vi "EOL Vent AP Test.vi"(7 "scaling factor":dbl=11.1, 10 "input cluster":T2 {"LIN INFO"."NAD" format="%.0x"; "LIN INFO"."ADCS LIN"."HW select" items=["NI-XNET", "NI-CAN"]; "LVDT Status"."LVDT's stored config"."Lower Limit" format="%.2f"; "LVDT Status"."LVDT's stored config"."Upper Limit" format="%.2f"; "PLC Comms"."PLC string write Tags"."error message 9"."DataSocket Reference"."OnStatusUpdated" format="%.0x"; "PLC Comms"."PLC string write Tags"."error message 9"."DataSocket Reference"."OnDataUpdated" format="%.0x"; "PLC Comms"."PLC string write Tags"."error message 8"."DataSocket Reference"."OnStatusUpdated" format="%.0x"; "PLC Comms"."PLC string write Tags"."error message 8"."DataSocket Reference"."OnDataUpdated" format="%.0x"; "PLC Comms"."PLC string write Tags"."error message 7"."DataSocket Reference"."OnStatusUpdated" format="%.0x"; "PLC Comms"."PLC string write Tags"."error message 7"."DataSocket Reference"."OnDataUpdated" format="%.0x"; "PLC Comms"."PLC string write Tags"."error message 6"."DataSocket Reference"."OnStatusUpdated" format="%.0x"; "PLC Comms"."PLC string write Tags"."error message 6"."DataSocket Reference"."OnDataUpdated" format="%.0x"; "PLC Comms"."PLC string write Tags"."error message 5"."DataSocket Reference"."OnStatusUpdated" format="%.0x"; "PLC Comms"."PLC string write Tags"."error message 5"."DataSocket Reference"."OnDataUpdated" format="%.0x"; "PLC Comms"."PLC string write Tags"."error message 4"."DataSocket Reference"."OnStatusUpdated" format="%.0x"; "PLC Comms"."PLC string write Tags"."error message 4"."DataSocket Reference"."OnDataUpdated" format="%.0x"; "PLC Comms"."PLC string write Tags"."error message 3"."DataSocket Reference"."OnStatusUpdated" format="%.0x"; "PLC Comms"."PLC string write Tags"."error message 3"."DataSocket Reference"."OnDataUpdated" format="%.0x"; "PLC Comms"."PLC string write Tags"."error message 2"."DataSocket Reference"."OnStatusUpdated" format="%.0x"; "PLC Comms"."PLC string write Tags"."error message 2"."DataSocket Reference"."OnDataUpdated" format="%.0x"; "PLC Comms"."PLC string write Tags"."error message 1"."DataSocket Reference"."OnStatusUpdated" format="%.0x"; "PLC Comms"."PLC string write Tags"."error message 1"."DataSocket Reference"."OnDataUpdated" format="%.0x"; "PLC Comms"."PLC string write Tags"."error message 0"."DataSocket Reference"."OnStatusUpdated" format="%.0x"; "PLC Comms"."PLC string write Tags"."error message 0"."DataSocket Reference"."OnDataUpdated" format="%.0x"; "PLC Comms"."PLC string write Tags"."barcode station error"."DataSocket Reference"."OnStatusUpdated" format="%.0x"; "PLC Comms"."PLC string write Tags"."barcode station error"."DataSocket Reference"."OnDataUpdated" format="%.0x"; "PLC Comms"."PLC string read Tags"."iGPS SN 9"."DataSocket Reference"."OnStatusUpdated" format="%.0x"; "PLC Comms"."PLC string read Tags"."iGPS SN 9"."DataSocket Reference"."OnDataUpdated" format="%.0x"; "PLC Comms"."PLC string read Tags"."iGPS SN 8"."DataSocket Reference"."OnStatusUpdated" format="%.0x"; "PLC Comms"."PLC string read Tags"."iGPS SN 8"."DataSocket Reference"."OnDataUpdated" format="%.0x"; "PLC Comms"."PLC string read Tags"."iGPS SN 7"."DataSocket Reference"."OnStatusUpdated" format="%.0x"; "PLC Comms"."PLC string read Tags"."iGPS SN 7"."DataSocket Reference"."OnDataUpdated" format="%.0x"; "PLC Comms"."PLC string read Tags"."iGPS SN 6"."DataSocket Reference"."OnStatusUpdated" format="%.0x"; "PLC Comms"."PLC string read Tags"."iGPS SN 6"."DataSocket Reference"."OnDataUpdated" format="%.0x"; "PLC Comms"."PLC string read Tags"."iGPS SN 5"."DataSocket Reference"."OnStatusUpdated" format="%.0x"; "PLC Comms"."PLC string read Tags"."iGPS SN 5"."DataSocket Reference"."OnDataUpdated" format="%.0x"; "PLC Comms"."PLC string read Tags"."iGPS SN 4"."DataSocket Reference"."OnStatusUpdated" format="%.0x"; "PLC Comms"."PLC string read Tags"."iGPS SN 4"."DataSocket Reference"."OnDataUpdated" format="%.0x"; "PLC Comms"."PLC string read Tags"."iGPS SN 3"."DataSocket Reference"."OnStatusUpdated" format="%.0x"; "PLC Comms"."PLC string read Tags"."iGPS SN 3"."DataSocket Reference"."OnDataUpdated" format="%.0x"; "PLC Comms"."PLC string read Tags"."iGPS SN 2"."DataSocket Reference"."OnStatusUpdated" format="%.0x"; "PLC Comms"."PLC string read Tags"."iGPS SN 2"."DataSocket Reference"."OnDataUpdated" format="%.0x"; "PLC Comms"."PLC string read Tags"."iGPS SN 1"."DataSocket Reference"."OnStatusUpdated" format="%.0x"; "PLC Comms"."PLC string read Tags"."iGPS SN 1"."DataSocket Reference"."OnDataUpdated" format="%.0x"; "PLC Comms"."PLC string read Tags"."iGPS SN 0"."DataSocket Reference"."OnStatusUpdated" format="%.0x"; "PLC Comms"."PLC string read Tags"."iGPS SN 0"."DataSocket Reference"."OnDataUpdated" format="%.0x"; "PLC Comms"."PLC string read Tags"."Manual Part History Number"."DataSocket Reference"."OnStatusUpdated" format="%.0x"; "PLC Comms"."PLC string read Tags"."Manual Part History Number"."DataSocket Reference"."OnDataUpdated" format="%.0x"; "PLC Comms"."PLC string read Tags"."Manual Customer Number"."DataSocket Reference"."OnStatusUpdated" format="%.0x"; "PLC Comms"."PLC string read Tags"."Manual Customer Number"."DataSocket Reference"."OnDataUpdated" format="%.0x"; "PLC Comms"."PLC string read Tags"."Manual Model Type"."DataSocket Reference"."OnStatusUpdated" format="%.0x"; "PLC Comms"."PLC string read Tags"."Manual Model Type"."DataSocket Reference"."OnDataUpdated" format="%.0x"; "PLC Comms"."PLC string read Tags"."Manual Shade Color"."DataSocket Reference"."OnStatusUpdated" format="%.0x"; "PLC Comms"."PLC string read Tags"."Manual Shade Color"."DataSocket Reference"."OnDataUpdated" format="%.0x"; "PLC Comms"."PLC string read Tags"."Manual Inalfa Part Number"."DataSocket Reference"."OnStatusUpdated" format="%.0x"; "PLC Comms"."PLC string read Tags"."Manual Inalfa Part Number"."DataSocket Reference"."OnDataUpdated" format="%.0x"; "PLC Comms"."PLC string read Tags"."Manual Serial Number"."DataSocket Reference"."OnStatusUpdated" format="%.0x"; "PLC Comms"."PLC string read Tags"."Manual Serial Number"."DataSocket Reference"."OnDataUpdated" format="%.0x"; "PLC Comms"."PLC string read Tags"."Shade 2 Barcode"."DataSocket Reference"."OnStatusUpdated" format="%.0x"; "PLC Comms"."PLC string read Tags"."Shade 2 Barcode"."DataSocket Reference"."OnDataUpdated" format="%.0x"; "PLC Comms"."PLC string read Tags"."Shade 1 Barcode"."DataSocket Reference"."OnStatusUpdated" format="%.0x"; "PLC Comms"."PLC string read Tags"."Shade 1 Barcode"."DataSocket Reference"."OnDataUpdated" format="%.0x"; "PLC Comms"."PLC string read Tags"."Part History Number"."DataSocket Reference"."OnStatusUpdated" format="%.0x"; "PLC Comms"."PLC string read Tags"."Part History Number"."DataSocket Reference"."OnDataUpdated" format="%.0x"; "PLC Comms"."PLC string read Tags"."Customer Number"."DataSocket Reference"."OnStatusUpdated" format="%.0x"; "PLC Comms"."PLC string read Tags"."Customer Number"."DataSocket Reference"."OnDataUpdated" format="%.0x"; "PLC Comms"."PLC string read Tags"."Model Type"."DataSocket Reference"."OnStatusUpdated" format="%.0x"; "PLC Comms"."PLC string read Tags"."Model Type"."DataSocket Reference"."OnDataUpdated" format="%.0x"; "PLC Comms"."PLC string read Tags"."Shade Color"."DataSocket Reference"."OnStatusUpdated" format="%.0x"; "PLC Comms"."PLC string read Tags"."Shade Color"."DataSocket Reference"."OnDataUpdated" format="%.0x"; "PLC Comms"."PLC string read Tags"."Inalfa Part Number"."DataSocket Reference"."OnStatusUpdated" format="%.0x"; "PLC Comms"."PLC string read Tags"."Inalfa Part Number"."DataSocket Reference"."OnDataUpdated" format="%.0x"; "PLC Comms"."PLC string read Tags"."Pallet Number"."DataSocket Reference"."OnStatusUpdated" format="%.0x"; "PLC Comms"."PLC string read Tags"."Pallet Number"."DataSocket Reference"."OnDataUpdated" format="%.0x"; "PLC Comms"."PLC string read Tags"."Serial Number"."DataSocket Reference"."OnStatusUpdated" format="%.0x"; "PLC Comms"."PLC string read Tags"."Serial Number"."DataSocket Reference"."OnDataUpdated" format="%.0x"; "PLC Comms"."PLC bool write Tags"."Move LVDT Adjust Station"."DataSocket Reference"."OnStatusUpdated" format="%.0x"; "PLC Comms"."PLC bool write Tags"."Move LVDT Adjust Station"."DataSocket Reference"."OnDataUpdated" format="%.0x"; "PLC Comms"."PLC bool write Tags"."AT set to Vent ATS Home Pos"."DataSocket Reference"."OnStatusUpdated" format="%.0x"; "PLC Comms"."PLC bool write Tags"."AT set to Vent ATS Home Pos"."DataSocket Reference"."OnDataUpdated" format="%.0x"; "PLC Comms"."PLC bool write Tags"."AT set to Vent ATS Test Pos"."DataSocket Reference"."OnStatusUpdated" format="%.0x"; "PLC Comms"."PLC bool write Tags"."AT set to Vent ATS Test Pos"."DataSocket Reference"."OnDataUpdated" format="%.0x"; "PLC Comms"."PLC bool write Tags"."Barcode02 OK"."DataSocket Reference"."OnStatusUpdated" format="%.0x"; "PLC Comms"."PLC bool write Tags"."Barcode02 OK"."DataSocket Reference"."OnDataUpdated" format="%.0x"; "PLC Comms"."PLC bool write Tags"."Barcode01 OK"."DataSocket Reference"."OnStatusUpdated" format="%.0x"; "PLC Comms"."PLC bool write Tags"."Barcode01 OK"."DataSocket Reference"."OnDataUpdated" format="%.0x"; "PLC Comms"."PLC bool write Tags"."AT set wand 02 home pos"."DataSocket Reference"."OnStatusUpdated" format="%.0x"; "PLC Comms"."PLC bool write Tags"."AT set wand 02 home pos"."DataSocket Reference"."OnDataUpdated" format="%.0x"; "PLC Comms"."PLC bool write Tags"."AT set sunshade 02 wand up"."DataSocket Reference"."OnStatusUpdated" format="%.0x"; "PLC Comms"."PLC bool write Tags"."AT set sunshade 02 wand up"."DataSocket Reference"."OnDataUpdated" format="%.0x"; "PLC Comms"."PLC bool write Tags"."NVH Operator Finish"."DataSocket Reference"."OnStatusUpdated" format="%.0x"; "PLC Comms"."PLC bool write Tags"."NVH Operator Finish"."DataSocket Reference"."OnDataUpdated" format="%.0x"; "PLC Comms"."PLC bool write Tags"."NVH Operator Glass Close Noise"."DataSocket Reference"."OnStatusUpdated" format="%.0x"; "PLC Comms"."PLC bool write Tags"."NVH Operator Glass Close Noise"."DataSocket Reference"."OnDataUpdated" format="%.0x"; "PLC Comms"."PLC bool write Tags"."NVH Operator Glass Open Noise"."DataSocket Reference"."OnStatusUpdated" format="%.0x"; "PLC Comms"."PLC bool write Tags"."NVH Operator Glass Open Noise"."DataSocket Reference"."OnDataUpdated" format="%.0x"; "PLC Comms"."PLC bool write Tags"."NVH Operator Sunshade Close Noise"."DataSocket Reference"."OnStatusUpdated" format="%.0x"; "PLC Comms"."PLC bool write Tags"."NVH Operator Sunshade Close Noise"."DataSocket Reference"."OnDataUpdated" format="%.0x"; "PLC Comms"."PLC bool write Tags"."NVH Operator Sunshade Open Noise"."DataSocket Reference"."OnStatusUpdated" format="%.0x"; "PLC Comms"."PLC bool write Tags"."NVH Operator Sunshade Open Noise"."DataSocket Reference"."OnDataUpdated" format="%.0x"; "PLC Comms"."PLC bool write Tags"."NVH Operator Vent Close Noise"."DataSocket Reference"."OnStatusUpdated" format="%.0x"; "PLC Comms"."PLC bool write Tags"."NVH Operator Vent Close Noise"."DataSocket Reference"."OnDataUpdated" format="%.0x"; "PLC Comms"."PLC bool write Tags"."NVH Operator Vent Open Noise"."DataSocket Reference"."OnStatusUpdated" format="%.0x"; "PLC Comms"."PLC bool write Tags"."NVH Operator Vent Open Noise"."DataSocket Reference"."OnDataUpdated" format="%.0x"; "PLC Comms"."PLC bool write Tags"."NVH Operator Check"."DataSocket Reference"."OnStatusUpdated" format="%.0x"; "PLC Comms"."PLC bool write Tags"."NVH Operator Check"."DataSocket Reference"."OnDataUpdated" format="%.0x"; "PLC Comms"."PLC bool write Tags"."NVH Operator Fail"."DataSocket Reference"."OnStatusUpdated" format="%.0x"; "PLC Comms"."PLC bool write Tags"."NVH Operator Fail"."DataSocket Reference"."OnDataUpdated" format="%.0x"; "PLC Comms"."PLC bool write Tags"."NVH Operator Pass"."DataSocket Reference"."OnStatusUpdated" format="%.0x"; "PLC Comms"."PLC bool write Tags"."NVH Operator Pass"."DataSocket Reference"."OnDataUpdated" format="%.0x"; "PLC Comms"."PLC bool write Tags"."NVH Operator Express Rollo Opened02"."DataSocket Reference"."OnStatusUpdated" format="%.0x"; "PLC Comms"."PLC bool write Tags"."NVH Operator Express Rollo Opened02"."DataSocket Reference"."OnDataUpdated" format="%.0x"; "PLC Comms"."PLC bool write Tags"."NVH Operator Express Rollo Closed01"."DataSocket Reference"."OnStatusUpdated" format="%.0x"; "PLC Comms"."PLC bool write Tags"."NVH Operator Express Rollo Closed01"."DataSocket Reference"."OnDataUpdated" format="%.0x"; "PLC Comms"."PLC bool write Tags"."NVH Operator Express Rollo Opened01"."DataSocket Reference"."OnStatusUpdated" format="%.0x"; "PLC Comms"."PLC bool write Tags"."NVH Operator Express Rollo Opened01"."DataSocket Reference"."OnDataUpdated" format="%.0x"; "PLC Comms"."PLC bool write Tags"."NVH Operator Express Glass Closed"."DataSocket Reference"."OnStatusUpdated" format="%.0x"; "PLC Comms"."PLC bool write Tags"."NVH Operator Express Glass Closed"."DataSocket Reference"."OnDataUpdated" format="%.0x"; "PLC Comms"."PLC bool write Tags"."NVH Operator Express Glass Opened"."DataSocket Reference"."OnStatusUpdated" format="%.0x"; "PLC Comms"."PLC bool write Tags"."NVH Operator Express Glass Opened"."DataSocket Reference"."OnDataUpdated" format="%.0x"; "PLC Comms"."PLC bool write Tags"."NVH Fail"."DataSocket Reference"."OnStatusUpdated" format="%.0x"; "PLC Comms"."PLC bool write Tags"."NVH Fail"."DataSocket Reference"."OnDataUpdated" format="%.0x"; "PLC Comms"."PLC bool write Tags"."NVH Pass"."DataSocket Reference"."OnStatusUpdated" format="%.0x"; "PLC Comms"."PLC bool write Tags"."NVH Pass"."DataSocket Reference"."OnDataUpdated" format="%.0x"; "PLC Comms"."PLC bool write Tags"."NVH SunRoof Stop"."DataSocket Reference"."OnStatusUpdated" format="%.0x"; "PLC Comms"."PLC bool write Tags"."NVH SunRoof Stop"."DataSocket Reference"."OnDataUpdated" format="%.0x"; "PLC Comms"."PLC bool write Tags"."NVH SunRoof Moving"."DataSocket Reference"."OnStatusUpdated" format="%.0x"; "PLC Comms"."PLC bool write Tags"."NVH SunRoof Moving"."DataSocket Reference"."OnDataUpdated" format="%.0x"; "PLC Comms"."PLC bool write Tags"."Extend Z LVDTS"."DataSocket Reference"."OnStatusUpdated" format="%.0x"; "PLC Comms"."PLC bool write Tags"."Extend Z LVDTS"."DataSocket Reference"."OnDataUpdated" format="%.0x"; "PLC Comms"."PLC bool write Tags"."Bad Frame Barcode"."DataSocket Reference"."OnStatusUpdated" format="%.0x"; "PLC Comms"."PLC bool write Tags"."Bad Frame Barcode"."DataSocket Reference"."OnDataUpdated" format="%.0x"; "PLC Comms"."PLC bool write Tags"."Good Frame Barcode"."DataSocket Reference"."OnStatusUpdated" format="%.0x"; "PLC Comms"."PLC bool write Tags"."Good Frame Barcode"."DataSocket Reference"."OnDataUpdated" format="%.0x"; "PLC Comms"."PLC bool write Tags"."AT VentPMACExtended"."DataSocket Reference"."OnStatusUpdated" format="%.0x"; "PLC Comms"."PLC bool write Tags"."AT VentPMACExtended"."DataSocket Reference"."OnDataUpdated" format="%.0x"; "PLC Comms"."PLC bool write Tags"."AT VentPMACHome"."DataSocket Reference"."OnStatusUpdated" format="%.0x"; "PLC Comms"."PLC bool write Tags"."AT VentPMACHome"."DataSocket Reference"."OnDataUpdated" format="%.0x"; "PLC Comms"."PLC bool write Tags"."control slide stop"."DataSocket Reference"."OnStatusUpdated" format="%.0x"; "PLC Comms"."PLC bool write Tags"."control slide stop"."DataSocket Reference"."OnDataUpdated" format="%.0x"; "PLC Comms"."PLC bool write Tags"."control slide start"."DataSocket Reference"."OnStatusUpdated" format="%.0x"; "PLC Comms"."PLC bool write Tags"."control slide start"."DataSocket Reference"."OnDataUpdated" format="%.0x"; "PLC Comms"."PLC bool write Tags"."ss servo close"."DataSocket Reference"."OnStatusUpdated" format="%.0x"; "PLC Comms"."PLC bool write Tags"."ss servo close"."DataSocket Reference"."OnDataUpdated" format="%.0x"; "PLC Comms"."PLC bool write Tags"."ss servo open"."DataSocket Reference"."OnStatusUpdated" format="%.0x"; "PLC Comms"."PLC bool write Tags"."ss servo open"."DataSocket Reference"."OnDataUpdated" format="%.0x"; "PLC Comms"."PLC bool write Tags"."Extend LVDT's"."DataSocket Reference"."OnStatusUpdated" format="%.0x"; "PLC Comms"."PLC bool write Tags"."Extend LVDT's"."DataSocket Reference"."OnDataUpdated" format="%.0x"; "PLC Comms"."PLC bool write Tags"."Retract LVDT's"."DataSocket Reference"."OnStatusUpdated" format="%.0x"; "PLC Comms"."PLC bool write Tags"."Retract LVDT's"."DataSocket Reference"."OnDataUpdated" format="%.0x"; "PLC Comms"."PLC bool write Tags"."Test Started"."DataSocket Reference"."OnStatusUpdated" format="%.0x"; "PLC Comms"."PLC bool write Tags"."Test Started"."DataSocket Reference"."OnDataUpdated" format="%.0x"; "PLC Comms"."PLC bool write Tags"."Test Complete Fail"."DataSocket Reference"."OnStatusUpdated" format="%.0x"; "PLC Comms"."PLC bool write Tags"."Test Complete Fail"."DataSocket Reference"."OnDataUpdated" format="%.0x"; "PLC Comms"."PLC bool write Tags"."Test Complete Pass"."DataSocket Reference"."OnStatusUpdated" format="%.0x"; "PLC Comms"."PLC bool write Tags"."Test Complete Pass"."DataSocket Reference"."OnDataUpdated" format="%.0x"; "PLC Comms"."PLC bool write Tags"."AT set wand home pos"."DataSocket Reference"."OnStatusUpdated" format="%.0x"; "PLC Comms"."PLC bool write Tags"."AT set wand home pos"."DataSocket Reference"."OnDataUpdated" format="%.0x"; "PLC Comms"."PLC bool write Tags"."AT set sunshade wand lower"."DataSocket Reference"."OnStatusUpdated" format="%.0x"; "PLC Comms"."PLC bool write Tags"."AT set sunshade wand lower"."DataSocket Reference"."OnDataUpdated" format="%.0x"; "PLC Comms"."PLC bool write Tags"."AT set glass wand lower"."DataSocket Reference"."OnStatusUpdated" format="%.0x"; "PLC Comms"."PLC bool write Tags"."AT set glass wand lower"."DataSocket Reference"."OnDataUpdated" format="%.0x"; "PLC Comms"."PLC boolean read Tags"."Finish Adjust LVDT"."DataSocket Reference"."OnStatusUpdated" format="%.0x"; "PLC Comms"."PLC boolean read Tags"."Finish Adjust LVDT"."DataSocket Reference"."OnDataUpdated" format="%.0x"; "PLC Comms"."PLC boolean read Tags"."Start Adjust LVDT"."DataSocket Reference"."OnStatusUpdated" format="%.0x"; "PLC Comms"."PLC boolean read Tags"."Start Adjust LVDT"."DataSocket Reference"."OnDataUpdated" format="%.0x"; "PLC Comms"."PLC boolean read Tags"."AT at vent ATS Home pos"."DataSocket Reference"."OnStatusUpdated" format="%.0x"; "PLC Comms"."PLC boolean read Tags"."AT at vent ATS Home pos"."DataSocket Reference"."OnDataUpdated" format="%.0x"; "PLC Comms"."PLC boolean read Tags"."AT at vent ATS test pos"."DataSocket Reference"."OnStatusUpdated" format="%.0x"; "PLC Comms"."PLC boolean read Tags"."AT at vent ATS test pos"."DataSocket Reference"."OnDataUpdated" format="%.0x"; "PLC Comms"."PLC boolean read Tags"."NVH Operator Re-do"."DataSocket Reference"."OnStatusUpdated" format="%.0x"; "PLC Comms"."PLC boolean read Tags"."NVH Operator Re-do"."DataSocket Reference"."OnDataUpdated" format="%.0x"; "PLC Comms"."PLC boolean read Tags"."NVH Operator Express Glass Vent Close"."DataSocket Reference"."OnStatusUpdated" format="%.0x"; "PLC Comms"."PLC boolean read Tags"."NVH Operator Express Glass Vent Close"."DataSocket Reference"."OnDataUpdated" format="%.0x"; "PLC Comms"."PLC boolean read Tags"."NVH Operator Express Glass vent Open"."DataSocket Reference"."OnStatusUpdated" format="%.0x"; "PLC Comms"."PLC boolean read Tags"."NVH Operator Express Glass vent Open"."DataSocket Reference"."OnDataUpdated" format="%.0x"; "PLC Comms"."PLC boolean read Tags"."windproof position"."DataSocket Reference"."OnStatusUpdated" format="%.0x"; "PLC Comms"."PLC boolean read Tags"."windproof position"."DataSocket Reference"."OnDataUpdated" format="%.0x"; "PLC Comms"."PLC boolean read Tags"."AT in wand 02 home pos"."DataSocket Reference"."OnStatusUpdated" format="%.0x"; "PLC Comms"."PLC boolean read Tags"."AT in wand 02 home pos"."DataSocket Reference"."OnDataUpdated" format="%.0x"; "PLC Comms"."PLC boolean read Tags"."AT in sunshad 02 wand up pos"."DataSocket Reference"."OnStatusUpdated" format="%.0x"; "PLC Comms"."PLC boolean read Tags"."AT in sunshad 02 wand up pos"."DataSocket Reference"."OnDataUpdated" format="%.0x"; "PLC Comms"."PLC boolean read Tags"."AT shade 02 position"."DataSocket Reference"."OnStatusUpdated" format="%.0x"; "PLC Comms"."PLC boolean read Tags"."AT shade 02 position"."DataSocket Reference"."OnDataUpdated" format="%.0x"; "PLC Comms"."PLC boolean read Tags"."NVH Operator Check"."DataSocket Reference"."OnStatusUpdated" format="%.0x"; "PLC Comms"."PLC boolean read Tags"."NVH Operator Check"."DataSocket Reference"."OnDataUpdated" format="%.0x"; "PLC Comms"."PLC boolean read Tags"."NVH Operator Finish"."DataSocket Reference"."OnStatusUpdated" format="%.0x"; "PLC Comms"."PLC boolean read Tags"."NVH Operator Finish"."DataSocket Reference"."OnDataUpdated" format="%.0x"; "PLC Comms"."PLC boolean read Tags"."NVH Operator Glass Close Noise"."DataSocket Reference"."OnStatusUpdated" format="%.0x"; "PLC Comms"."PLC boolean read Tags"."NVH Operator Glass Close Noise"."DataSocket Reference"."OnDataUpdated" format="%.0x"; "PLC Comms"."PLC boolean read Tags"."NVH Operator Glass Open Noise"."DataSocket Reference"."OnStatusUpdated" format="%.0x"; "PLC Comms"."PLC boolean read Tags"."NVH Operator Glass Open Noise"."DataSocket Reference"."OnDataUpdated" format="%.0x"; "PLC Comms"."PLC boolean read Tags"."NVH Operator Sunshade Close Noise"."DataSocket Reference"."OnStatusUpdated" format="%.0x"; "PLC Comms"."PLC boolean read Tags"."NVH Operator Sunshade Close Noise"."DataSocket Reference"."OnDataUpdated" format="%.0x"; "PLC Comms"."PLC boolean read Tags"."NVH Operator Sunshade Open Noise"."DataSocket Reference"."OnStatusUpdated" format="%.0x"; "PLC Comms"."PLC boolean read Tags"."NVH Operator Sunshade Open Noise"."DataSocket Reference"."OnDataUpdated" format="%.0x"; "PLC Comms"."PLC boolean read Tags"."NVH Operator Vent Close Noise"."DataSocket Reference"."OnStatusUpdated" format="%.0x"; "PLC Comms"."PLC boolean read Tags"."NVH Operator Vent Close Noise"."DataSocket Reference"."OnDataUpdated" format="%.0x"; "PLC Comms"."PLC boolean read Tags"."NVH Operator Vent Open Noise"."DataSocket Reference"."OnStatusUpdated" format="%.0x"; "PLC Comms"."PLC boolean read Tags"."NVH Operator Vent Open Noise"."DataSocket Reference"."OnDataUpdated" format="%.0x"; "PLC Comms"."PLC boolean read Tags"."NVH Operator Express Rollo Close02"."DataSocket Reference"."OnStatusUpdated" format="%.0x"; "PLC Comms"."PLC boolean read Tags"."NVH Operator Express Rollo Close02"."DataSocket Reference"."OnDataUpdated" format="%.0x"; "PLC Comms"."PLC boolean read Tags"."NVH Operator Express Rollo Open02"."DataSocket Reference"."OnStatusUpdated" format="%.0x"; "PLC Comms"."PLC boolean read Tags"."NVH Operator Express Rollo Open02"."DataSocket Reference"."OnDataUpdated" format="%.0x"; "PLC Comms"."PLC boolean read Tags"."NVH Operator Express Rollo Close01"."DataSocket Reference"."OnStatusUpdated" format="%.0x"; "PLC Comms"."PLC boolean read Tags"."NVH Operator Express Rollo Close01"."DataSocket Reference"."OnDataUpdated" format="%.0x"; "PLC Comms"."PLC boolean read Tags"."NVH Operator Express Rollo Open01"."DataSocket Reference"."OnStatusUpdated" format="%.0x"; "PLC Comms"."PLC boolean read Tags"."NVH Operator Express Rollo Open01"."DataSocket Reference"."OnDataUpdated" format="%.0x"; "PLC Comms"."PLC boolean read Tags"."NVH Operator Express Glass Close"."DataSocket Reference"."OnStatusUpdated" format="%.0x"; "PLC Comms"."PLC boolean read Tags"."NVH Operator Express Glass Close"."DataSocket Reference"."OnDataUpdated" format="%.0x"; "PLC Comms"."PLC boolean read Tags"."NVH Operator Express Glass Open"."DataSocket Reference"."OnStatusUpdated" format="%.0x"; "PLC Comms"."PLC boolean read Tags"."NVH Operator Express Glass Open"."DataSocket Reference"."OnDataUpdated" format="%.0x"; "PLC Comms"."PLC boolean read Tags"."NVH Operator Fail"."DataSocket Reference"."OnStatusUpdated" format="%.0x"; "PLC Comms"."PLC boolean read Tags"."NVH Operator Fail"."DataSocket Reference"."OnDataUpdated" format="%.0x"; "PLC Comms"."PLC boolean read Tags"."NVH Operator Pass"."DataSocket Reference"."OnStatusUpdated" format="%.0x"; "PLC Comms"."PLC boolean read Tags"."NVH Operator Pass"."DataSocket Reference"."OnDataUpdated" format="%.0x"; "PLC Comms"."PLC boolean read Tags"."Z LVDTs Extended"."DataSocket Reference"."OnStatusUpdated" format="%.0x"; "PLC Comms"."PLC boolean read Tags"."Z LVDTs Extended"."DataSocket Reference"."OnDataUpdated" format="%.0x"; "PLC Comms"."PLC boolean read Tags"."iGPS Pass 9"."DataSocket Reference"."OnStatusUpdated" format="%.0x"; "PLC Comms"."PLC boolean read Tags"."iGPS Pass 9"."DataSocket Reference"."OnDataUpdated" format="%.0x"; "PLC Comms"."PLC boolean read Tags"."iGPS Pass 8"."DataSocket Reference"."OnStatusUpdated" format="%.0x"; "PLC Comms"."PLC boolean read Tags"."iGPS Pass 8"."DataSocket Reference"."OnDataUpdated" format="%.0x"; "PLC Comms"."PLC boolean read Tags"."iGPS Pass 7"."DataSocket Reference"."OnStatusUpdated" format="%.0x"; "PLC Comms"."PLC boolean read Tags"."iGPS Pass 7"."DataSocket Reference"."OnDataUpdated" format="%.0x"; "PLC Comms"."PLC boolean read Tags"."iGPS Pass 6"."DataSocket Reference"."OnStatusUpdated" format="%.0x"; "PLC Comms"."PLC boolean read Tags"."iGPS Pass 6"."DataSocket Reference"."OnDataUpdated" format="%.0x"; "PLC Comms"."PLC boolean read Tags"."iGPS Pass 5"."DataSocket Reference"."OnStatusUpdated" format="%.0x"; "PLC Comms"."PLC boolean read Tags"."iGPS Pass 5"."DataSocket Reference"."OnDataUpdated" format="%.0x"; "PLC Comms"."PLC boolean read Tags"."iGPS Pass 4"."DataSocket Reference"."OnStatusUpdated" format="%.0x"; "PLC Comms"."PLC boolean read Tags"."iGPS Pass 4"."DataSocket Reference"."OnDataUpdated" format="%.0x"; "PLC Comms"."PLC boolean read Tags"."iGPS Pass 3"."DataSocket Reference"."OnStatusUpdated" format="%.0x"; "PLC Comms"."PLC boolean read Tags"."iGPS Pass 3"."DataSocket Reference"."OnDataUpdated" format="%.0x"; "PLC Comms"."PLC boolean read Tags"."iGPS Pass 2"."DataSocket Reference"."OnStatusUpdated" format="%.0x"; "PLC Comms"."PLC boolean read Tags"."iGPS Pass 2"."DataSocket Reference"."OnDataUpdated" format="%.0x"; "PLC Comms"."PLC boolean read Tags"."iGPS Pass 1"."DataSocket Reference"."OnStatusUpdated" format="%.0x"; "PLC Comms"."PLC boolean read Tags"."iGPS Pass 1"."DataSocket Reference"."OnDataUpdated" format="%.0x"; "PLC Comms"."PLC boolean read Tags"."iGPS Pass 0"."DataSocket Reference"."OnStatusUpdated" format="%.0x"; "PLC Comms"."PLC boolean read Tags"."iGPS Pass 0"."DataSocket Reference"."OnDataUpdated" format="%.0x"; "PLC Comms"."PLC boolean read Tags"."Check Frame Barcode"."DataSocket Reference"."OnStatusUpdated" format="%.0x"; "PLC Comms"."PLC boolean read Tags"."Check Frame Barcode"."DataSocket Reference"."OnDataUpdated" format="%.0x"; "PLC Comms"."PLC boolean read Tags"."SS Barcode Scanner Bypassed"."DataSocket Reference"."OnStatusUpdated" format="%.0x"; "PLC Comms"."PLC boolean read Tags"."SS Barcode Scanner Bypassed"."DataSocket Reference"."OnDataUpdated" format="%.0x"; "PLC Comms"."PLC boolean read Tags"."AT VentPMACisExtend"."DataSocket Reference"."OnStatusUpdated" format="%.0x"; "PLC Comms"."PLC boolean read Tags"."AT VentPMACisExtend"."DataSocket Reference"."OnDataUpdated" format="%.0x"; "PLC Comms"."PLC boolean read Tags"."AT VentPMACatHome"."DataSocket Reference"."OnStatusUpdated" format="%.0x"; "PLC Comms"."PLC boolean read Tags"."AT VentPMACatHome"."DataSocket Reference"."OnDataUpdated" format="%.0x"; "PLC Comms"."PLC boolean read Tags"."wind deflector low speed pos"."DataSocket Reference"."OnStatusUpdated" format="%.0x"; "PLC Comms"."PLC boolean read Tags"."wind deflector low speed pos"."DataSocket Reference"."OnDataUpdated" format="%.0x"; "PLC Comms"."PLC boolean read Tags"."wind deflector high speed pos"."DataSocket Reference"."OnStatusUpdated" format="%.0x"; "PLC Comms"."PLC boolean read Tags"."wind deflector high speed pos"."DataSocket Reference"."OnDataUpdated" format="%.0x"; "PLC Comms"."PLC boolean read Tags"."control slide right over stroke"."DataSocket Reference"."OnStatusUpdated" format="%.0x"; "PLC Comms"."PLC boolean read Tags"."control slide right over stroke"."DataSocket Reference"."OnDataUpdated" format="%.0x"; "PLC Comms"."PLC boolean read Tags"."control slide right good"."DataSocket Reference"."OnStatusUpdated" format="%.0x"; "PLC Comms"."PLC boolean read Tags"."control slide right good"."DataSocket Reference"."OnDataUpdated" format="%.0x"; "PLC Comms"."PLC boolean read Tags"."control slide left over stroke"."DataSocket Reference"."OnStatusUpdated" format="%.0x"; "PLC Comms"."PLC boolean read Tags"."control slide left over stroke"."DataSocket Reference"."OnDataUpdated" format="%.0x"; "PLC Comms"."PLC boolean read Tags"."control slide left good"."DataSocket Reference"."OnStatusUpdated" format="%.0x"; "PLC Comms"."PLC boolean read Tags"."control slide left good"."DataSocket Reference"."OnDataUpdated" format="%.0x"; "PLC Comms"."PLC boolean read Tags"."control slide at home"."DataSocket Reference"."OnStatusUpdated" format="%.0x"; "PLC Comms"."PLC boolean read Tags"."control slide at home"."DataSocket Reference"."OnDataUpdated" format="%.0x"; "PLC Comms"."PLC boolean read Tags"."ss servo closing"."DataSocket Reference"."OnStatusUpdated" format="%.0x"; "PLC Comms"."PLC boolean read Tags"."ss servo closing"."DataSocket Reference"."OnDataUpdated" format="%.0x"; "PLC Comms"."PLC boolean read Tags"."ss servo opening"."DataSocket Reference"."OnStatusUpdated" format="%.0x"; "PLC Comms"."PLC boolean read Tags"."ss servo opening"."DataSocket Reference"."OnDataUpdated" format="%.0x"; "PLC Comms"."PLC boolean read Tags"."ss servo at close"."DataSocket Reference"."OnStatusUpdated" format="%.0x"; "PLC Comms"."PLC boolean read Tags"."ss servo at close"."DataSocket Reference"."OnDataUpdated" format="%.0x"; "PLC Comms"."PLC boolean read Tags"."ss servo at open"."DataSocket Reference"."OnStatusUpdated" format="%.0x"; "PLC Comms"."PLC boolean read Tags"."ss servo at open"."DataSocket Reference"."OnDataUpdated" format="%.0x"; "PLC Comms"."PLC boolean read Tags"."manual barcode print"."DataSocket Reference"."OnStatusUpdated" format="%.0x"; "PLC Comms"."PLC boolean read Tags"."manual barcode print"."DataSocket Reference"."OnDataUpdated" format="%.0x"; "PLC Comms"."PLC boolean read Tags"."LVDT's Retracted"."DataSocket Reference"."OnStatusUpdated" format="%.0x"; "PLC Comms"."PLC boolean read Tags"."LVDT's Retracted"."DataSocket Reference"."OnDataUpdated" format="%.0x"; "PLC Comms"."PLC boolean read Tags"."abort"."DataSocket Reference"."OnStatusUpdated" format="%.0x"; "PLC Comms"."PLC boolean read Tags"."abort"."DataSocket Reference"."OnDataUpdated" format="%.0x"; "PLC Comms"."PLC boolean read Tags"."start"."DataSocket Reference"."OnStatusUpdated" format="%.0x"; "PLC Comms"."PLC boolean read Tags"."start"."DataSocket Reference"."OnDataUpdated" format="%.0x"; "PLC Comms"."PLC boolean read Tags"."bolt check 21"."DataSocket Reference"."OnStatusUpdated" format="%.0x"; "PLC Comms"."PLC boolean read Tags"."bolt check 21"."DataSocket Reference"."OnDataUpdated" format="%.0x"; "PLC Comms"."PLC boolean read Tags"."bolt check 20"."DataSocket Reference"."OnStatusUpdated" format="%.0x"; "PLC Comms"."PLC boolean read Tags"."bolt check 20"."DataSocket Reference"."OnDataUpdated" format="%.0x"; "PLC Comms"."PLC boolean read Tags"."bolt check 19"."DataSocket Reference"."OnStatusUpdated" format="%.0x"; "PLC Comms"."PLC boolean read Tags"."bolt check 19"."DataSocket Reference"."OnDataUpdated" format="%.0x"; "PLC Comms"."PLC boolean read Tags"."bolt check 18"."DataSocket Reference"."OnStatusUpdated" format="%.0x"; "PLC Comms"."PLC boolean read Tags"."bolt check 18"."DataSocket Reference"."OnDataUpdated" format="%.0x"; "PLC Comms"."PLC boolean read Tags"."bolt check 17"."DataSocket Reference"."OnStatusUpdated" format="%.0x"; "PLC Comms"."PLC boolean read Tags"."bolt check 17"."DataSocket Reference"."OnDataUpdated" format="%.0x"; "PLC Comms"."PLC boolean read Tags"."bolt check 16"."DataSocket Reference"."OnStatusUpdated" format="%.0x"; "PLC Comms"."PLC boolean read Tags"."bolt check 16"."DataSocket Reference"."OnDataUpdated" format="%.0x"; "PLC Comms"."PLC boolean read Tags"."bolt check 15"."DataSocket Reference"."OnStatusUpdated" format="%.0x"; "PLC Comms"."PLC boolean read Tags"."bolt check 15"."DataSocket Reference"."OnDataUpdated" format="%.0x"; "PLC Comms"."PLC boolean read Tags"."bolt check 14"."DataSocket Reference"."OnStatusUpdated" format="%.0x"; "PLC Comms"."PLC boolean read Tags"."bolt check 14"."DataSocket Reference"."OnDataUpdated" format="%.0x"; "PLC Comms"."PLC boolean read Tags"."bolt check 13"."DataSocket Reference"."OnStatusUpdated" format="%.0x"; "PLC Comms"."PLC boolean read Tags"."bolt check 13"."DataSocket Reference"."OnDataUpdated" format="%.0x"; "PLC Comms"."PLC boolean read Tags"."bolt check 12"."DataSocket Reference"."OnStatusUpdated" format="%.0x"; "PLC Comms"."PLC boolean read Tags"."bolt check 12"."DataSocket Reference"."OnDataUpdated" format="%.0x"; "PLC Comms"."PLC boolean read Tags"."bolt check 11"."DataSocket Reference"."OnStatusUpdated" format="%.0x"; "PLC Comms"."PLC boolean read Tags"."bolt check 11"."DataSocket Reference"."OnDataUpdated" format="%.0x"; "PLC Comms"."PLC boolean read Tags"."bolt check 10"."DataSocket Reference"."OnStatusUpdated" format="%.0x"; "PLC Comms"."PLC boolean read Tags"."bolt check 10"."DataSocket Reference"."OnDataUpdated" format="%.0x"; "PLC Comms"."PLC boolean read Tags"."bolt check 9"."DataSocket Reference"."OnStatusUpdated" format="%.0x"; "PLC Comms"."PLC boolean read Tags"."bolt check 9"."DataSocket Reference"."OnDataUpdated" format="%.0x"; "PLC Comms"."PLC boolean read Tags"."bolt check 8"."DataSocket Reference"."OnStatusUpdated" format="%.0x"; "PLC Comms"."PLC boolean read Tags"."bolt check 8"."DataSocket Reference"."OnDataUpdated" format="%.0x"; "PLC Comms"."PLC boolean read Tags"."bolt check 7"."DataSocket Reference"."OnStatusUpdated" format="%.0x"; "PLC Comms"."PLC boolean read Tags"."bolt check 7"."DataSocket Reference"."OnDataUpdated" format="%.0x"; "PLC Comms"."PLC boolean read Tags"."bolt check 6"."DataSocket Reference"."OnStatusUpdated" format="%.0x"; "PLC Comms"."PLC boolean read Tags"."bolt check 6"."DataSocket Reference"."OnDataUpdated" format="%.0x"; "PLC Comms"."PLC boolean read Tags"."bolt check 5"."DataSocket Reference"."OnStatusUpdated" format="%.0x"; "PLC Comms"."PLC boolean read Tags"."bolt check 5"."DataSocket Reference"."OnDataUpdated" format="%.0x"; "PLC Comms"."PLC boolean read Tags"."bolt check 4"."DataSocket Reference"."OnStatusUpdated" format="%.0x"; "PLC Comms"."PLC boolean read Tags"."bolt check 4"."DataSocket Reference"."OnDataUpdated" format="%.0x"; "PLC Comms"."PLC boolean read Tags"."bolt check 3"."DataSocket Reference"."OnStatusUpdated" format="%.0x"; "PLC Comms"."PLC boolean read Tags"."bolt check 3"."DataSocket Reference"."OnDataUpdated" format="%.0x"; "PLC Comms"."PLC boolean read Tags"."bolt check 2"."DataSocket Reference"."OnStatusUpdated" format="%.0x"; "PLC Comms"."PLC boolean read Tags"."bolt check 2"."DataSocket Reference"."OnDataUpdated" format="%.0x"; "PLC Comms"."PLC boolean read Tags"."bolt check 1"."DataSocket Reference"."OnStatusUpdated" format="%.0x"; "PLC Comms"."PLC boolean read Tags"."bolt check 1"."DataSocket Reference"."OnDataUpdated" format="%.0x"; "PLC Comms"."PLC boolean read Tags"."FB light block present"."DataSocket Reference"."OnStatusUpdated" format="%.0x"; "PLC Comms"."PLC boolean read Tags"."FB light block present"."DataSocket Reference"."OnDataUpdated" format="%.0x"; "PLC Comms"."PLC boolean read Tags"."audit gap hider present RH"."DataSocket Reference"."OnStatusUpdated" format="%.0x"; "PLC Comms"."PLC boolean read Tags"."audit gap hider present RH"."DataSocket Reference"."OnDataUpdated" format="%.0x"; "PLC Comms"."PLC boolean read Tags"."audit gap hider present LH"."DataSocket Reference"."OnStatusUpdated" format="%.0x"; "PLC Comms"."PLC boolean read Tags"."audit gap hider present LH"."DataSocket Reference"."OnDataUpdated" format="%.0x"; "PLC Comms"."PLC boolean read Tags"."motor foam present RH"."DataSocket Reference"."OnStatusUpdated" format="%.0x"; "PLC Comms"."PLC boolean read Tags"."motor foam present RH"."DataSocket Reference"."OnDataUpdated" format="%.0x"; "PLC Comms"."PLC boolean read Tags"."motor foam present LH"."DataSocket Reference"."OnStatusUpdated" format="%.0x"; "PLC Comms"."PLC boolean read Tags"."motor foam present LH"."DataSocket Reference"."OnDataUpdated" format="%.0x"; "PLC Comms"."PLC boolean read Tags"."LVDT's Extended"."DataSocket Reference"."OnStatusUpdated" format="%.0x"; "PLC Comms"."PLC boolean read Tags"."LVDT's Extended"."DataSocket Reference"."OnDataUpdated" format="%.0x"; "PLC Comms"."PLC boolean read Tags"."AT in wand home pos"."DataSocket Reference"."OnStatusUpdated" format="%.0x"; "PLC Comms"."PLC boolean read Tags"."AT in wand home pos"."DataSocket Reference"."OnDataUpdated" format="%.0x"; "PLC Comms"."PLC boolean read Tags"."AT in sunshad wand lower pos"."DataSocket Reference"."OnStatusUpdated" format="%.0x"; "PLC Comms"."PLC boolean read Tags"."AT in sunshad wand lower pos"."DataSocket Reference"."OnDataUpdated" format="%.0x"; "PLC Comms"."PLC boolean read Tags"."AT in glass wand lower pos"."DataSocket Reference"."OnStatusUpdated" format="%.0x"; "PLC Comms"."PLC boolean read Tags"."AT in glass wand lower pos"."DataSocket Reference"."OnDataUpdated" format="%.0x"; "PLC Comms"."PLC boolean read Tags"."AT shade position"."DataSocket Reference"."OnStatusUpdated" format="%.0x"; "PLC Comms"."PLC boolean read Tags"."AT shade position"."DataSocket Reference"."OnDataUpdated" format="%.0x"; "PLC Comms"."PLC boolean read Tags"."AT glass position"."DataSocket Reference"."OnStatusUpdated" format="%.0x"; "PLC Comms"."PLC boolean read Tags"."AT glass position"."DataSocket Reference"."OnDataUpdated" format="%.0x"; "Store Data"."Sun Shade Open Force Limits"."Variance" format="%.2g"; "Store Data"."Sun Shade Open Force Limits"."Truncation End" format="%.2g"; "Store Data"."Sun Shade Open Force Limits"."Truncation Start" format="%.2g"; "Store Data"."Sun Shade Open Force Limits"."Avg Max" format="%.2g"; "Store Data"."Sun Shade Open Force Limits"."Avg Min" format="%.2g"; "Store Data"."Sun Shade Open Force Limits"."Overall Max" format="%.2g"; "Store Data"."Sun Shade Open Force Limits"."Overall Min" format="%.2g"; "Store Data"."Sun Shade Close Force Limits"."Variance" format="%.2g"; "Store Data"."Sun Shade Close Force Limits"."Truncation End" format="%.2g"; "Store Data"."Sun Shade Close Force Limits"."Truncation Start" format="%.2g"; "Store Data"."Sun Shade Close Force Limits"."Avg Max" format="%.2g"; "Store Data"."Sun Shade Close Force Limits"."Avg Min" format="%.2g"; "Store Data"."Sun Shade Close Force Limits"."Overall Max" format="%.2g"; "Store Data"."Sun Shade Close Force Limits"."Overall Min" format="%.2g"}) -> (0 "Error Table Out":string[][](array[string]), 1 "Vent Force Raw Data":sgl[](graph), 2 "Vent Force Data and Limits":dbl[](array[numeric]), 3 "Pass? Out":bool, 5 "Sun Shade Close Force":T1 {"Truncation End" format="%.2g"; "Truncation Start" format="%.2g"; "Overall Max" format="%.2g"; "Overall Min" format="%.2g"})   [LabVIEW 2018]
uses:
  02.Type Def's/EOL Analog Input Control.ctl
  05.UserVI's/type defs/Vent AP Limts Seq.ctl
  05.UserVI's/type defs/17x Sunshade Limts Seq.ctl
  05.UserVI's/type defs/plc path and tag.ctl
  02.Type Def's/station plc write boolean tags.ctl
  02.Type Def's/station plc read boolean tags.ctl
  05.UserVI's/type defs/EOL Motor Type.ctl
  05.UserVI's/type defs/RAP Signal Control.ctl
  05.UserVI's/type defs/Communication with Motors.ctl
  02.Type Def's/All Communication Types.ctl
  05.UserVI's/type defs/EOL Part Setup.ctl
  02.Type Def's/All Motions.ctl
  02.Type Def's/EOL Switch Max Min Check Cluster.ctl
  02.Type Def's/EOL Switch Value Configuration Cluster.ctl
  02.Type Def's/All Switch Configuration Cluster.ctl
  02.Type Def's/Pass Fail Control.ctl
  02.Type Def's/EOL Module Info Control.ctl
  05.UserVI's/type defs/17x AP Data Type.ctl
  05.UserVI's/type defs/17x Audit Motion Data Seq Control.ctl
  02.Type Def's/EOL Motion Database Table.ctl
  05.UserVI's/sequence/type defs/Sequence Info.ctl
  02.Type Def's/station nvh config.ctl
  05.UserVI's/type defs/EOL Global Digital Output Control.ctl
  02.Type Def's/station DO map.ctl
  02.Type Def's/station rs232 port map.ctl
  02.Type Def's/station ethernet address map.ctl
  02.Type Def's/station paths.ctl
  02.Type Def's/EOL Save Module Test Data Control.ctl
  05.UserVI's/type defs/EOL Global Digital Input Control.ctl
  02.Type Def's/station DI map.ctl
  02.Type Def's/station plc read string tags.ctl
  02.Type Def's/station plc write string tags.ctl
  02.Type Def's/Screen Motion Data.ctl
  02.Type Def's/station motion data indicator.ctl
  02.Type Def's/lvdt name val pair.ctl
  02.Type Def's/station hmi.ctl
  02.Type Def's/individual station status.ctl
  02.Type Def's/control refs.ctl
  05.UserVI's/Lambda Power/power supply types.ctl
  02.Type Def's/main state cluster.ctl
  <vilib>/Platform/dataskt.llb/DataSocket Reference Type.ctl
  05.UserVI's/type defs/EOL LVDT's Check Controller.ctl
  05.UserVI's/LVDT's/lvdt precision.ctl
  02.Type Def's/station plc read float tags.ctl
  02.Type Def's/plc comms params.ctl
  02.Type Def's/iGPS float tags.ctl
  02.Type Def's/sequence state.ctl
  03.Inalfa LIN/LIN Device.ctl
  <vilib>/CMC.AME/Inalfa ADCS/Ctl'Def/ADCS_LIN info.ctl
  C:/Program Files (x86)/National Instruments/LabVIEW 2018/vi.lib/CMC.AME/_Inalfa TS LIN_internal_deps/Interop.TSMasterAPI.dll
  Program Files (x86)/National Instruments/LabVIEW 2018/vi.lib/CMC.AME/_Inalfa TS LIN_internal_deps/Interop.TSMasterAPI.dll
  02.Type Def's/station LIN config.ctl
  02.Type Def's/misc station config.ctl
panel:
  out "State":string
  # "Start"
  # "Min"
  # "N"
  # "End"
  # "Max"
  # "N"
  # "start/abort only used by barcode instance, since there are discrete signals for this in the other stations."
  # "Sunroof Barcode"
  # "Pallet Number"
  # "Part Type"
  # "Application Status"
  # "Current Step"
  # "Cycle Time"
  # "Pass / Fail"
  # "Shade Close"
  # "Actual Data"
  # "Limits"
  # "Avg Current"
  # "Run Time"
  # "Speed"
  # "Noise Test"
  # "Position"
  # "Shade Open"
  # "Actual Data"
  # "Limits"
  # "Avg Current"
  # "Run Time"
  # "Speed"
  # "Noise Test"
  # "Position"
  # "Vent Close"
  # "Actual Data"
  # "Limits"
  # "Avg Current"
  # "Run Time"
  # "Speed"
  # "Noise Test"
  # "Position"
  # "Vent Open"
  # "Actual Data"
  # "Limits"
  # "Avg Current"
  # "Run Time"
  # "Speed"
  # "Noise Test"
  # "Position"
  # "Slide Close"
  # "Actual Data"
  # "Limits"
  # "Avg Current"
  # "Run Time"
  # "Speed"
  # "Noise Test"
  # "Position"
  # "Slide Open"
  # "Actual Data"
  # "Limits"
  # "Avg Current"
  # "Run Time"
  # "Speed"
  # "Noise Test"
  # "Position"
  # "Min"
  # "N"
  # "Min"
  # "Start"
  # "N"
  # "Max"
  # "N"
  # "Max"
  # "N"
  # "End"
  # "Min"
  # "N"
  # "Min"
  # "Start"
  # "N"
  # "Max"
  # "N"
  # "Max"
  # "N"
  # "End"
  # "Min"
  # "Max"
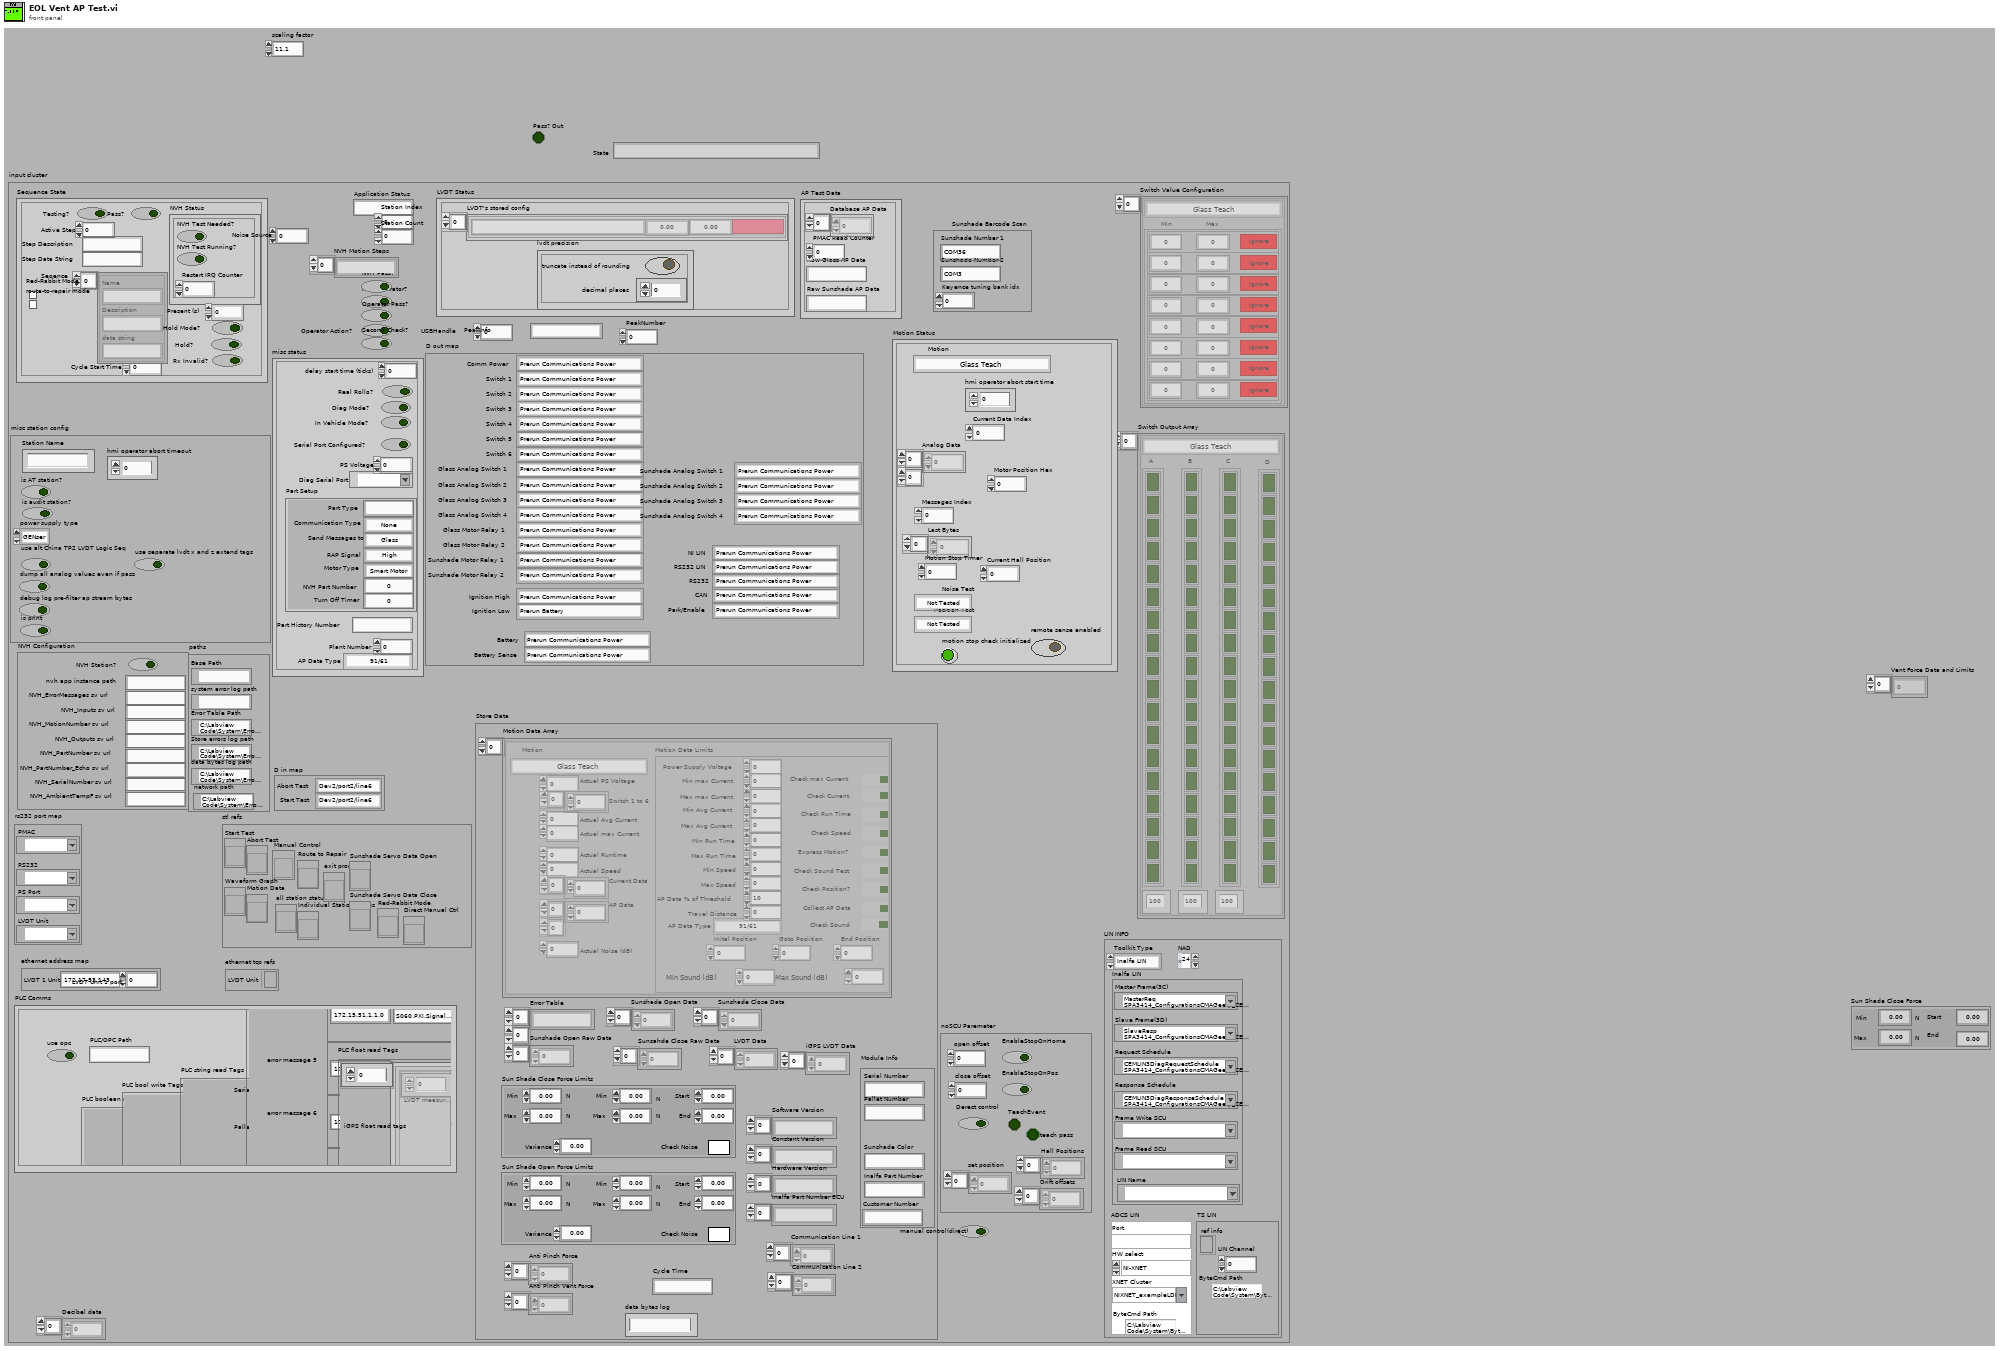
[diagram p1: front panel]
types:
  T1 = typedef "Vent AP Limts Seq.ctl" = cluster{"Overall Min":dbl, "Overall Max":dbl, "Truncation Start":dbl, "Truncation End":dbl}
  T2 = typedef "main state cluster.ctl" = cluster{"Application Status":string, "Switch Output Array":T3[], "Switch Value Configuration":T5[], "NVH Configuration":T7, "D out map":T8, "rs232 port map":T10, "ethernet address map":T11, "paths":T12, "Station Index":i32, "Station Count":i32, "Store Data":T13, "D in map":T19, "ctl refs":T21, "misc station config":T22, "ethernet tcp refs":cluster{"LVDT Unit":refnum<k5>}, "PLC Comms":T24, "Sunshade Barcode Scan":cluster{"Sunshade Number 2":string, "Sunshade Number 1":string, "Keyence tuning bank idx":i32}, "AP Test Data":cluster{"Raw Sunshade AP Data":string, "Raw Glass AP Data":string, "PMAC Read Counter":dbl, "Database AP Data":dbl[]}, "Motion Status":cluster{"hmi operator abort start time":u32, "Current Data Index":i32, "Analog Data":sgl[][], "Motor Position Hex":u16, "Messages Index":u16, "Last Bytes":u8[], "Current Hall Position":i16, "Motion Stop Timer":u32, "Position Test":T33, "Noise Test":T33, "motion stop check initialized":bool, "remote sense enabled":bool, "Motion":T4}, "LVDT Status":cluster{"LVDT's stored config":T34[], "lvdt precision":T35}, "Sequence State":T36, "misc status":cluster{"delay start time (ticks)":u32, "In Vehicle Mode?":bool, "Diag Mode?":bool, "Serial Port Configured?":bool, "PS Voltage":dbl, "Diag Serial Port":refnum<visa-resource-name>, "Part Setup":T38, "Part History Number":string, "Plant Number":u8, "AP Data Type":T16, "Real Rollo?":bool}, "NVH Operator?":bool, "NVH Pass?":bool, "Operator Pass?":bool, "Operator Action?":bool, "Noise Source":u32, "USBHandle":i32, "PeakInfo":string, "PeakNumber":i32, "NVH Motion Steps":string[], "Second Check?":bool, "Decibel data":dbl[], "noSCU Paremeter":cluster{"EnableStopOnHome":bool, "EnableStopOnPos":bool, "TeachEvent":bool, "open offset":i32, "close offset":i32, "Derect control":bool, "set position":i32[], "teach pass ":bool, "Drift offsets":i32[], "Hall Positions":i32[]}, "manual control(direct)":bool, "LIN INFO":T43}
  T3 = typedef "All Switch Configuration Cluster.ctl" = cluster{"All Motions":T4, "A":bool[], "B":bool[], "C":bool[], "D":bool[], "A activation time (ms)":u32, "B activation time (ms)":u32, "C activation time (ms)":u32}
  T4 = typedef "All Motions.ctl" = enum16{"Glass Teach", "Glass Slide Open", "Glass Slide Close", "Glass Vent Open", "Glass Vent Close", "Sunshade Teach", "Sunshade Open", "Sunshade Close", "Idle", "Sunshade Open 2", "Sunshade Close 2", "Glass Slide Open Sunshade Open", "Glass Slide Open Sunshade Close", "Glass Slide Close Sunshade Open", "Glass Slide Close Sunshade Close", "Glass Vent Open Sunshade Open", "Glass Vent Open Sunshade Close", "Glass Vent Close Sunshade Open", "Glass Vent Close Sunshade Close", "Express Glass Slide Open", "Express Glass Slide Close", "Express Glass Vent Open", "Express Glass Vent Close", "Express Sunshade Open", "Express Sunshade Close", "Express Sunshade Open 2", "Express Sunshade Close 2", "Express Glass Slide Open Sunshade Open", "Express Glass Slide Open Sunshade Close", "Express Glass Slide Close Sunshade Open", "Express Glass Slide Close Sunshade Close", "Express Glass Vent Open Sunshade Open", "Express Glass Vent Open Sunshade Close", "Express Glass Vent Close Sunshade Open", "Express Glass Vent Close Sunshade Close", "Goto Position Glass", "Goto Position Sunshade", "Sunshade Teach 2"}
  T5 = typedef "EOL Switch Value Configuration Cluster.ctl" = cluster{"All Motions":T4, "Array":T6[]}
  T6 = typedef "EOL Switch Max Min Check Cluster.ctl" = cluster{"Min":dbl, "Max":dbl, "Check?":bool}
  T7 = typedef "station nvh config.ctl" = cluster{"NVH Station?":bool, "nvh app instance path":string, "NVH_ErrorMessages sv url":string, "NVH_Inputs sv url":string, "NVH_MotionNumber sv url":string, "NVH_Outputs sv url":string, "NVH_PartNumber sv url":string, "NVH_PartNumber_Echo sv url":string, "NVH_SerialNumber sv url":string, "NVH_AmbientTempF sv url":string}
  T8 = typedef "station DO map.ctl" = cluster{"Comm Power":T9, "Switch 1":T9, "Switch 2":T9, "Switch 3":T9, "Switch 4":T9, "Switch 5":T9, "Switch 6":T9, "Glass Analog Switch 1":T9, "Glass Analog Switch 2":T9, "Glass Analog Switch 3":T9, "Glass Analog Switch 4":T9, "Glass Motor Relay 1":T9, "Glass Motor Relay 2":T9, "Sunshade Motor Relay 1":T9, "Sunshade Motor Relay 2":T9, "Ignition High":T9, "Ignition Low":T9, "Battery":T9, "Sunshade Analog Switch 1":T9, "Sunshade Analog Switch 2":T9, "Sunshade Analog Switch 3":T9, "Sunshade Analog Switch 4":T9, "NI LIN":T9, "RS232 LIN":T9, "RS232":T9, "CAN":T9, "Park/Enable":T9, "Battery Sense":T9}
  T9 = typedef "EOL Global Digital Output Control.ctl" = enum16{"Prerun Battery", "Prerun Ignition High", "Prerun Switch 1", "Prerun Switch 2", "Prerun Switch 3", "Prerun Select NI LIN", "Prerun Switch 4", "Prerun Switch 5", "Prerun Switch 6", "Prerun Ignition Low", "Prerun Glass Analog Switch 1", "Prerun Glass Analog Switch 2", "Prerun Glass Analog Switch 3", "Prerun Glass Analog Switch 4", "Prerun Sunshade Analog Switch 1", "Prerun Sunshade Analog Switch 2", "Prerun Sunshade Analog Switch 3", "Prerun Sunshade Analog Switch 4", "Prerun Select RS232 LIN", "Prerun Select RS232", "Prerun Select CAN", "Prerun Park/Enable", "Prerun Communications Power", "Prerun BMW Glass Motor Relay 1", "Prerun BMW Glass Motor Relay 2", "Prerun BMW Sunshade Motor Relay 1", "Prerun BMW Sunshade Motor Relay 2", "Prerun Spare 1", "Prerun Spare 2", "Prerun Spare 3", "Prerun Spare 4", "Prerun Spare 5", "Audit Battery", "Audit Ignition High", "Audit Ignition Low", "Audit Switch 1", "Audit Switch 2", "Audit Switch 3", "Audit Switch 4", "Audit Switch 5", "Audit Switch 6", "Audit Glass Analog Switch 1", "Audit Glass Analog Switch 2", "Audit Glass Analog Switch 3", "Audit Glass Analog Switch 4", "Audit Sunshade Analog Switch 1", "Audit Sunshade Analog Switch 2", "Audit Sunshade Analog Switch 3", "Audit Sunshade Analog Switch 4", "Audit Select NI LIN", "Audit Select RS232 LIN", "Audit Select RS232", "Audit Select CAN", "Audit Park/Enable", "Audit Communications Power", "Audit BMW Glass Motor Relay 1", "Audit BMW Glass Motor Relay 2", "Audit BMW Sunshade Motor Relay 1", "Audit BMW Sunshade Motor Relay 2", "Audit Spare 1", "Audit Spare 2", "Audit Spare 3", "Audit Spare 4", "Audit Spare 5", "Repair Battery", "Repair Ignition High", "Repair Switch 1", "Repair Switch 2", "Repair Select NI LIN", "Repair Ignition Low", "Repair Switch 3", "Repair Switch 4", "Repair Switch 5", "Repair Switch 6", "Repair Glass Analog Switch 1", "Repair Glass Analog Switch 2", "Repair Glass Analog Switch 3", "Repair Glass Analog Switch 4", "Repair Sunshade Analog Switch 1", "Repair Sunshade Analog Switch 2", "Repair Sunshade Analog Switch 3", "Repair Sunshade Analog Switch 4", "Repair Select RS232 LIN", "Repair Select RS232", "Repair Select CAN", "Repair Select Park/Enable", "Repair Communications Power", "Repair BMW Glass Motor Relay 1", "Repair BMW Glass Motor Relay 2", "Repair BMW Sunshade Motor Relay 1", "Repair BMW Sunshade Motor Relay 2", "Repair Spare 1", "Repair Spare 2", "Repair Spare 3", "Repair Spare 4", "Repair Spare 5", "Breakin Battery", "Breakin Igntiion High", "Breakin Ignition Low", "Breakin Switch 1", "Breakin Switch 2", "Breakin Switch 3", "Breakin Switch 4", "Breakin Switch 5", "Breakin Switch 6", "Breakin Glass Analog Switch 1", "Breakin Glass Analog Switch 2", "Breakin Glass Analog Switch 3", "Breakin Glass Analog Switch 4", "Breakin Sunshade Analog Switch 1", "Breakin Sunshade Analog Switch 2", "Breakin Sunshade Analog Switch 3", "Breakin Sunshade Analog Switch 4", "Breakin Select NI LIN", "Breakin Select RS232 LIN", "Breakin Select RS232", "Breakin Select CAN", "Breakin Park/Enable", "Breakin Communications Power", "Breakin BMW Glass Motor Relay 1", "Breakin BMW Glass Motor Relay 2", "Breakin BMW Sunshade Motor Relay 1", "Breakin BMW Sunshade Motor Relay 2", "Breakin Spare 1", "Breakin Spare 2", "Breakin Spare 3", "Breakin Spare 4", "Breakin Spare 5", "Not Implemented"}
  T10 = typedef "station rs232 port map.ctl" = cluster{"PMAC":refnum<visa-resource-name>, "PS Port":refnum<visa-resource-name>, "LVDT Unit":refnum<visa-resource-name>, "RS232":refnum<visa-resource-name>}
  T11 = typedef "station ethernet address map.ctl" = cluster{"LVDT 1 Unit":string, "LVDT Unit 1 port":u16}
  T12 = typedef "station paths.ctl" = cluster{"Base Path":path, "system error log path":path, "Error Table Path":path, "Store errors log path":path, "data bytes log path":path, "network path":path}
  T13 = typedef "EOL Save Module Test Data Control.ctl" = cluster{"Motion Data Array":T14[], "Error Table":string[][], "Sun Shade Close Force Limits":T17, "Sun Shade Open Force Limits":T17, "Sunshade Open Data":sgl[], "Sunshade Close Data":sgl[], "Module Info":T18, "Sunsahde Close Raw Data":sgl[], "Sunshade Open Raw Data":sgl[], "Software Version":string[], "Constant Version":string[], "Hardware Version":string[], "Inalfa Part Number ECU":string[], "LVDT Data":sgl[], "Communication Line 1":sgl[], "Communication Line 2":sgl[], "Anti Pinch Force":sgl[], "Cycle Time":string, "Anti Pinch Vent Force":sgl[], "iGPS LVDT Data":sgl[], "data bytes log":string}
  T14 = typedef "EOL Motion Database Table.ctl" = cluster{"Motion":T4, "Actual Avg Current":dbl, "Actual Runtime":dbl, "Actual Speed":dbl, "Current Data":sgl[], "Motion Data Limits":T15, "Switch 1 to 6":dbl[], "Actual PS Voltage":dbl, "AP Data":i16[][], "Actual max Current":dbl, "Actual Noise (dB)":dbl}
  T15 = typedef "17x Audit Motion Data Seq Control.ctl" = cluster{"Power Supply Voltage":dbl, "Min Avg Current":dbl, "Max Avg Current":dbl, "Min Run Time":dbl, "Max Run Time":dbl, "Min Speed":dbl, "Max Speed":dbl, "AP Data % of Threshold":dbl, "Travel Distance":dbl, "AP Data Type":T16, "Check Current":bool, "Check Run Time":bool, "Check Speed":bool, "Express Motion?":bool, "Check Sound Test":bool, "Check Position?":bool, "Collect AP Data":bool, "Inital Position":u16, "End Position":u16, "Goto Posiition":u16, "Max max Current":dbl, "Min max Current":dbl, "Check max Current":bool, "Check Sound":bool, "Min Sound (dB)":dbl, "Max Sound (dB)":dbl}
  T16 = typedef "17x AP Data Type.ctl" = enum16{"91/61", "92/62", "93/63", "67", "68", "6F", "71", "91 Msg", "92 Msg", "93 Msg", "94 Msg", "HiRain 91", "HiRain 92 Speed", "HiRain 92 HS", "HiRain 92", "HiRain 93", "SnT"}
  T17 = typedef "17x Sunshade Limts Seq.ctl" = cluster{"Overall Min":dbl, "Overall Max":dbl, "Avg Min":dbl, "Avg Max":dbl, "Truncation Start":dbl, "Truncation End":dbl, "Variance":dbl, "Check Noise":bool}
  T18 = typedef "EOL Module Info Control.ctl" = cluster{"Serial Number":string, "Pallet Number":string, "Sunshade Color":string, "Inalfa Part Number":string, "Customer Number":string}
  T19 = typedef "station DI map.ctl" = cluster{"Abort Test":T20, "Start Test":T20}
  T20 = typedef "EOL Global Digital Input Control.ctl" = enum16{"Dev2/port0/line0", "Dev2/port0/line1", "Dev2/port0/line2", "Dev2/port0/line3", "Dev2/port0/line4", "Dev2/port0/line5", "Dev2/port0/line6", "Dev2/port0/line7", "Dev2/port1/line0", "Dev2/port1/line1", "Dev2/port1/line2", "Dev2/port1/line3", "Dev2/port1/line4", "Dev2/port1/line5", "Dev2/port1/line6", "Dev2/port1/line7", "Dev2/port2/line0", "Dev2/port2/line1", "Dev2/port2/line2", "Dev2/port2/line3", "Dev2/port2/line4", "Dev2/port2/line5", "Dev2/port2/line6", "Dev2/port2/line7", "Prerun Start Test", "Prerun Abort Test", "Audit Start Test", "Audit Abort Test", "Dev2/port3/line4", "Dev2/port3/line5", "Breakin Start Test", "Breakin Abort Test", "Not Implemented"}
  T21 = typedef "control refs.ctl" = cluster{"Start Test":refnum<vi>, "Abort Test":refnum<vi>, "Manual Control":refnum<vi>, "Route to Repair":refnum<vi>, "Waveform Graph":refnum<vi>, "Motion Data":refnum<vi>, "all station status":refnum<vi>, "Individual Station Status":refnum<vi>, "exit program":refnum<vi>, "Sunshade Servo Data Open":refnum<vi>, "Sunshade Servo Data Close":refnum<vi>, "Red-Rabbit Mode":refnum<vi>, "Direct Manual Ctrl":refnum<vi>}
  T22 = typedef "misc station config.ctl" = cluster{"Station Name":string, "is AT station?":bool, "is audit station?":bool, "power supply type":T23, "use alt China TP2 LVDT Logic Seq":bool, "hmi operator abort timeout":u32, "dump all analog values even if pass":bool, "debug log pre-filter ap stream bytes":bool, "use separate lvdt x and z extend tags":bool, "is print":bool}
  T23 = typedef "power supply types.ctl" = enum16{"GENser", "ZUPser", "GENeth", "Manual", "ITECH"}
  T24 = typedef "plc comms params.ctl" = cluster{"PLC boolean read Tags":T25, "PLC bool write Tags":T28, "PLC string read Tags":T29, "PLC string write Tags":T30, "use opc":bool, "PLC/OPC Path":string, "PLC float read Tags":T31}
  T25 = typedef "station plc read boolean tags.ctl" = cluster{"AT glass position":T26, "AT shade position":T26, "AT in glass wand lower pos":T26, "AT in sunshad wand lower pos":T26, "AT in wand home pos":T26, "LVDT's Extended":T26, "motor foam present LH":T26, "motor foam present RH":T26, "audit gap hider present LH":T26, "audit gap hider present RH":T26, "FB light block present":T26, "bolt check 1":T26, "bolt check 2":T26, "bolt check 3":T26, "bolt check 4":T26, "bolt check 5":T26, "bolt check 6":T26, "bolt check 7":T26, "bolt check 8":T26, "bolt check 9":T26, "bolt check 10":T26, "bolt check 11":T26, "bolt check 12":T26, "bolt check 13":T26, "bolt check 14":T26, "bolt check 15":T26, "bolt check 16":T26, "bolt check 17":T26, "bolt check 18":T26, "bolt check 19":T26, "bolt check 20":T26, "bolt check 21":T26, "start":T26, "abort":T26, "LVDT's Retracted":T26, "manual barcode print":T26, "ss servo at open":T26, "ss servo at close":T26, "ss servo opening":T26, "ss servo closing":T26, "control slide at home":T26, "control slide left good":T26, "control slide left over stroke":T26, "control slide right good":T26, "control slide right over stroke":T26, "wind deflector high speed pos":T26, "wind deflector low speed pos":T26, "AT VentPMACatHome":T26, "AT VentPMACisExtend":T26, "SS Barcode Scanner Bypassed":T26, "Check Frame Barcode":T26, "iGPS Pass 0":T26, "iGPS Pass 1":T26, "iGPS Pass 2":T26, "iGPS Pass 3":T26, "iGPS Pass 4":T26, "iGPS Pass 5":T26, "iGPS Pass 6":T26, "iGPS Pass 7":T26, "iGPS Pass 8":T26, "iGPS Pass 9":T26, "Z LVDTs Extended":T26, "NVH Operator Pass":T26, "NVH Operator Fail":T26, "NVH Operator Express Glass Open":T26, "NVH Operator Express Glass Close":T26, "NVH Operator Express Rollo Open01":T26, "NVH Operator Express Rollo Close01":T26, "NVH Operator Express Rollo Open02":T26, "NVH Operator Express Rollo Close02":T26, "NVH Operator Vent Open Noise":T26, "NVH Operator Vent Close Noise":T26, "NVH Operator Sunshade Open Noise":T26, "NVH Operator Sunshade Close Noise":T26, "NVH Operator Glass Open Noise":T26, "NVH Operator Glass Close Noise":T26, "NVH Operator Finish":T26, "NVH Operator Check":T26, "AT shade 02 position":T26, "AT in sunshad 02 wand up pos":T26, "AT in wand 02 home pos":T26, "windproof position":T26, "NVH Operator Express Glass vent Open":T26, "NVH Operator Express Glass Vent Close":T26, "NVH Operator Re-do":T26, "AT at vent ATS test pos":T26, "AT at vent ATS Home pos":T26, "Start Adjust LVDT":T26, "Finish Adjust LVDT":T26}
  T26 = typedef "plc path and tag.ctl" = cluster{"Tag Name":string, "Network Path":string, "use opc":bool, "DataSocket Reference":T27}
  T27 = typedef "DataSocket Reference Type.ctl" = cluster{"CWDSLib._DCWDataSocket":refnum<k7>, "CWDSLib._DCWData":refnum<k7>, "OnDataUpdated":u32, "OnStatusUpdated":u32}
  T28 = typedef "station plc write boolean tags.ctl" = cluster{"AT set glass wand lower":T26, "AT set sunshade wand lower":T26, "AT set wand home pos":T26, "Test Complete Pass":T26, "Test Complete Fail":T26, "Test Started":T26, "Retract LVDT's":T26, "Extend LVDT's":T26, "ss servo open":T26, "ss servo close":T26, "control slide start":T26, "control slide stop":T26, "AT VentPMACHome":T26, "AT VentPMACExtended":T26, "Good Frame Barcode":T26, "Bad Frame Barcode":T26, "Extend Z LVDTS":T26, "NVH SunRoof Moving":T26, "NVH SunRoof Stop":T26, "NVH Pass":T26, "NVH Fail":T26, "NVH Operator Express Glass Opened":T26, "NVH Operator Express Glass Closed":T26, "NVH Operator Express Rollo Opened01":T26, "NVH Operator Express Rollo Closed01":T26, "NVH Operator Express Rollo Opened02":T26, "NVH Operator Pass":T26, "NVH Operator Fail":T26, "NVH Operator Check":T26, "NVH Operator Vent Open Noise":T26, "NVH Operator Vent Close Noise":T26, "NVH Operator Sunshade Open Noise":T26, "NVH Operator Sunshade Close Noise":T26, "NVH Operator Glass Open Noise":T26, "NVH Operator Glass Close Noise":T26, "NVH Operator Finish":T26, "AT set sunshade 02 wand up":T26, "AT set wand 02 home pos":T26, "Barcode01 OK":T26, "Barcode02 OK":T26, "AT set to Vent ATS Test Pos":T26, "AT set to Vent ATS Home Pos":T26, "Move LVDT Adjust Station":T26}
  T29 = typedef "station plc read string tags.ctl" = cluster{"Serial Number":T26, "Pallet Number":T26, "Inalfa Part Number":T26, "Shade Color":T26, "Model Type":T26, "Customer Number":T26, "Part History Number":T26, "Shade 1 Barcode":T26, "Shade 2 Barcode":T26, "Manual Serial Number":T26, "Manual Inalfa Part Number":T26, "Manual Shade Color":T26, "Manual Model Type":T26, "Manual Customer Number":T26, "Manual Part History Number":T26, "iGPS SN 0":T26, "iGPS SN 1":T26, "iGPS SN 2":T26, "iGPS SN 3":T26, "iGPS SN 4":T26, "iGPS SN 5":T26, "iGPS SN 6":T26, "iGPS SN 7":T26, "iGPS SN 8":T26, "iGPS SN 9":T26}
  T30 = typedef "station plc write string tags.ctl" = cluster{"barcode station error":T26, "error message 0":T26, "error message 1":T26, "error message 2":T26, "error message 3":T26, "error message 4":T26, "error message 5":T26, "error message 6":T26, "error message 7":T26, "error message 8":T26, "error message 9":T26}
  T31 = typedef "station plc read float tags.ctl" = cluster{"iGPS float read tags":T32[]}
  T32 = typedef "iGPS float tags.ctl" = cluster{"LVDT measurements":cluster{"value":T26, "UCL":T26, "LCL":T26, "LVDT Name":string}[]}
  T33 = typedef "Pass Fail Control.ctl" = enum16{"Not Tested", "Pass", "Fail"}
  T34 = typedef "EOL LVDT's Check Controller.ctl" = cluster{"Upper Limit":dbl, "Lower Limit":dbl, "LVDT Name":string, "Check":bool}
  T35 = typedef "lvdt precision.ctl" = cluster{"truncate instead of rounding":bool, "decimal places":u8}
  T36 = typedef "sequence state.ctl" = cluster{"Step Description":string, "Cycle Start Time":u32, "Step Data String":string, "Pass?":bool, "Seqence":T37[], "Active Step":u8, "Testing?":bool, "Red-Rabbit Mode":bool, "route-to-repair mode":bool, "NVH Status":cluster{"Restart IRQ Counter":u8, "NVH Test Needed?":bool, "NVH Test Running?":bool}, "Present (s)":dbl, "Hold Mode?":bool, "Hold?":bool, "Rx Invalid?":bool}
  T37 = typedef "Sequence Info.ctl" = cluster{"Name":string, "Description":string, "data string":string}
  T38 = typedef "EOL Part Setup.ctl" = cluster{"Communication Type":T39, "Send Messages to":T40, "RAP Signal":T41, "Motor Type":T42, "NVH Part Number":u16, "Turn Off Timer":u16, "Part Type":string}
  T39 = typedef "All Communication Types.ctl" = enum16{"None", "CAN", "RS 232", "RS 232 LIN", "GM LIN", "SnT LIN", "K Line", "Robel CAN", "P42M-Continental", "Inalfa SCU LIN", "Spare 3"}
  T40 = typedef "Communication with Motors.ctl" = enum16{"Glass", "Rollo", "Both"}
  T41 = typedef "RAP Signal Control.ctl" = enum16{"High", "Low", "None"}
  T42 = typedef "EOL Motor Type.ctl" = enum16{"Smart Motor", "Sensor Motor"}
  T43 = typedef "station LIN config.ctl" = cluster{"Toolkit Type":enum16{"Inalfa LIN", "ADCS LIN", "TS LIN"}, "NAD":u8, "Inalfa LIN":T44, "ADCS LIN":T45, "TS LIN":cluster{"ref info":refnum<k24>, "LIN Channel":i32, "ByteCmd Path":path}}
  T44 = typedef "LIN Device.ctl" = cluster{"Master Frame(3C)":refnum<k21>, "Slave Frame(3D)":refnum<k21>, "Request Schedule":refnum<k21>, "Response Schedule":refnum<k21>, "Frame Write SCU":refnum<k21>, "Frame Read SCU":refnum<k21>, "LIN Name":refnum<k21>}
  T45 = typedef "ADCS_LIN info.ctl" = cluster{"Port":string, "HW select":u16, "XNET Cluster":string, "ByteCmd Path":path}
  T46 = cluster{"Error String Array":string[], "Error String Number":u16[], "Vent Force Raw Data":sgl[], "Sun Shade Close Force":T1, "Pass?":bool, "Error Table":string[][], "Vent Force calculated data":dbl, "Station Index":i32, "PLC boolean read Tags":T25, "PLC bool write Tags":T28, "Abort Test":T20, "Vent Force Data and Limits":dbl[], "Analog Data":sgl[][]}
  T47 = typedef "EOL Analog Input Control.ctl" = enum16{"SW PS  Volage", "SW IGN Bat", "Switch A", "Switch B", "Motor Voltage", "Motor Current", "SW LIN", "ATS", "External ECU Current"}
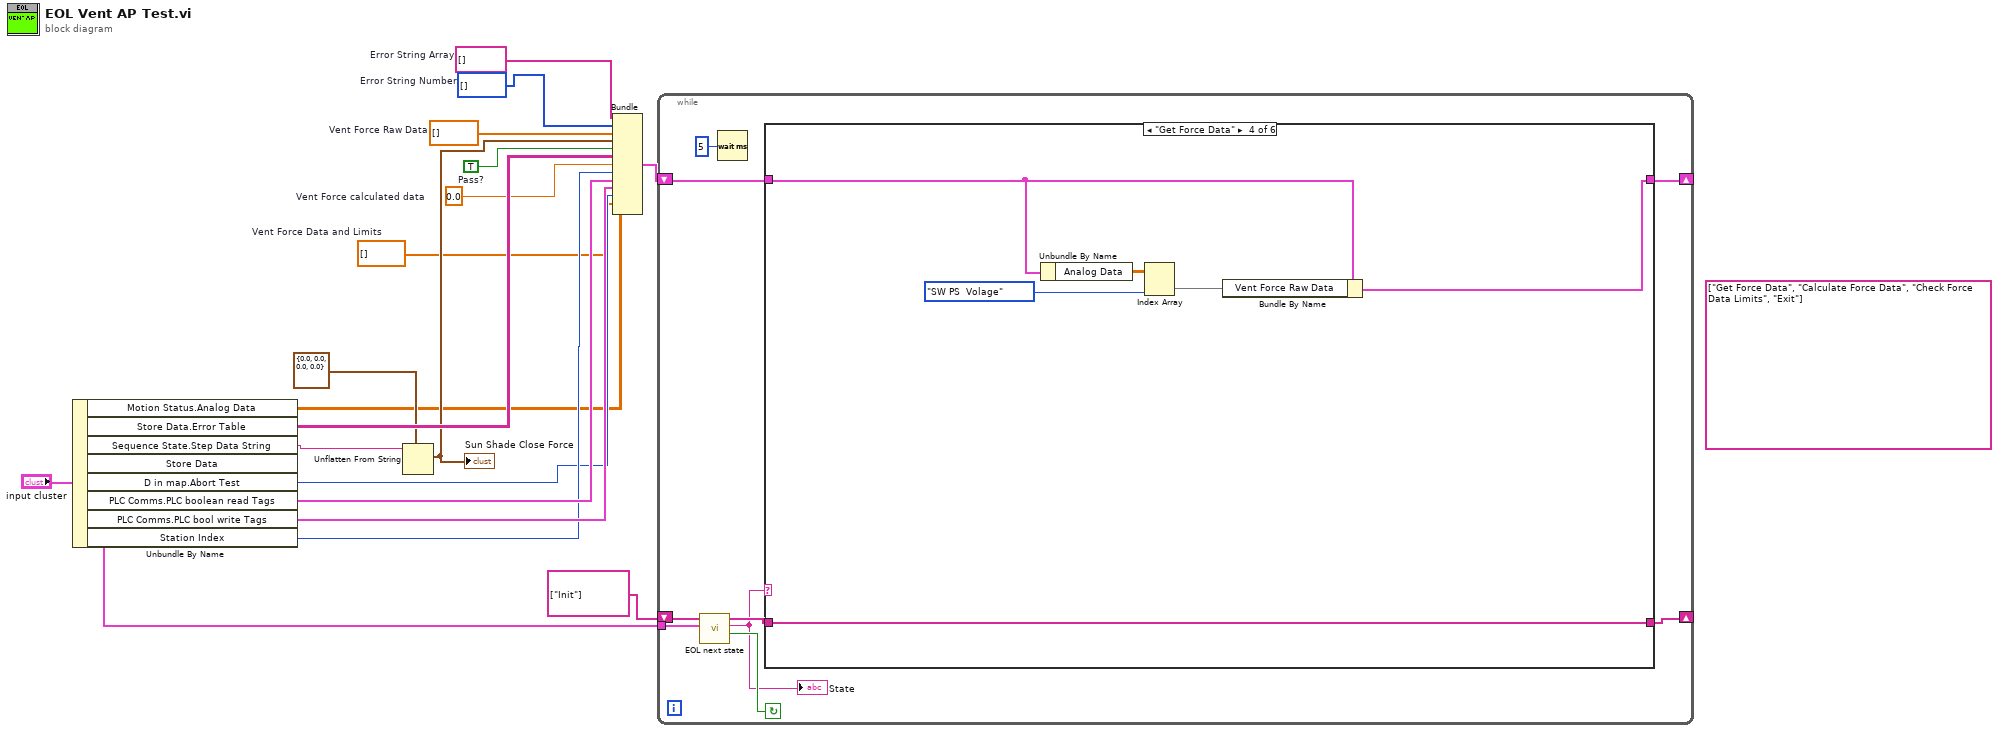
[diagram p0: block diagram]
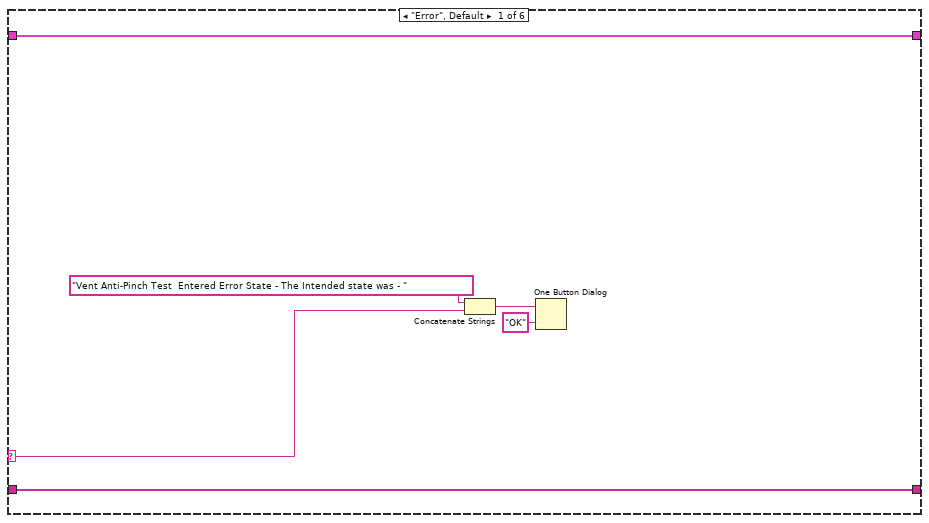
[diagram p2: hidden frame]
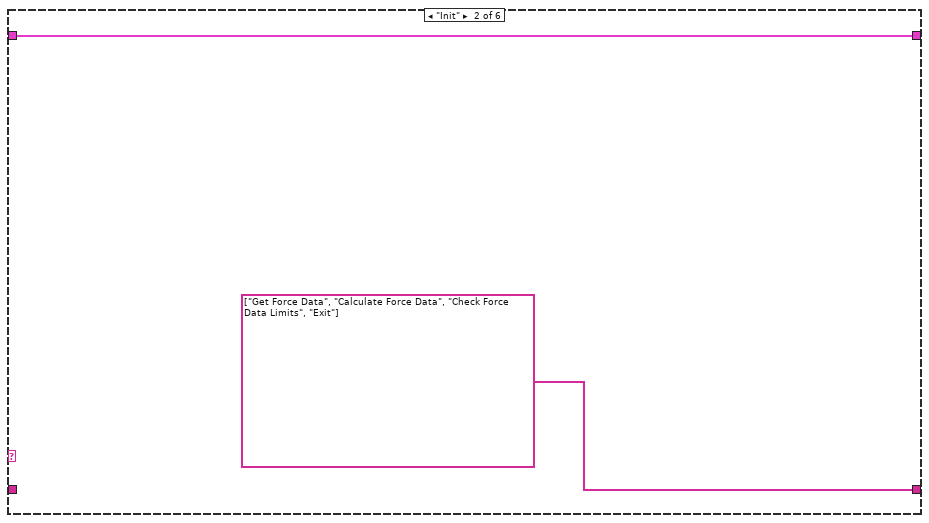
[diagram p3: hidden frame]
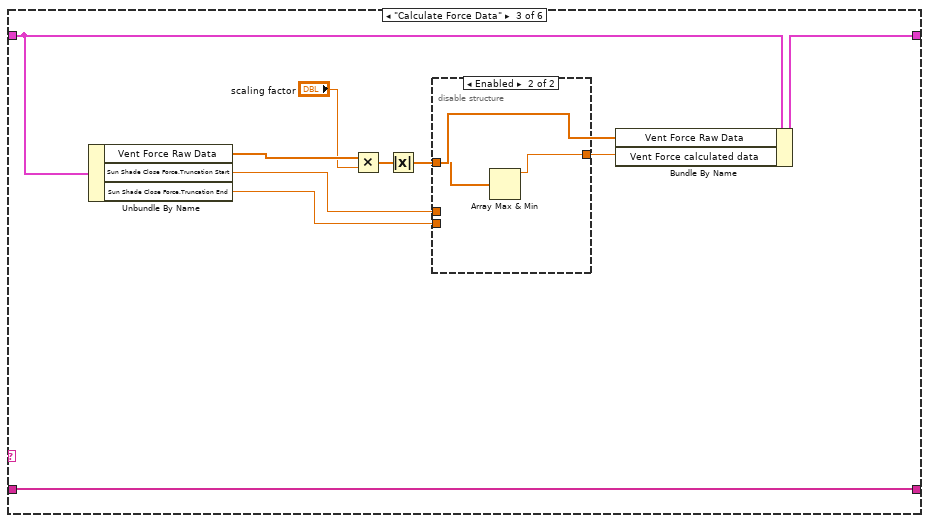
[diagram p4: hidden frame]
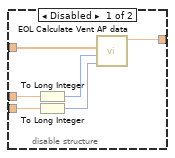
[diagram p5: hidden frame]
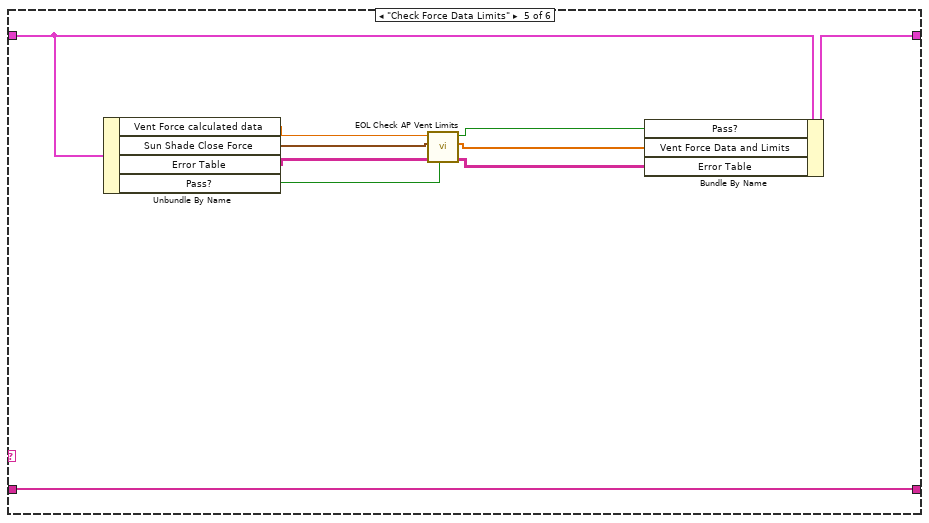
[diagram p6: hidden frame]
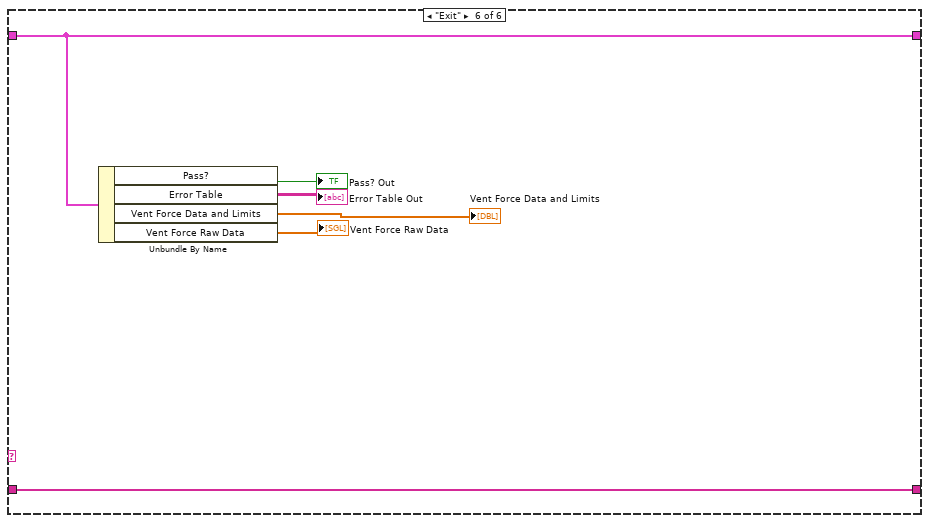
[diagram p7: hidden frame]
diagram:
  (unwired) string[] ["Get Force Data", "Calculate Force Data", "Check Force Data Limits", "Exit"] ("event queue out")
  w2 = dbl[] []  # Vent Force Data and Limits
  w3 = 0.0  # Vent Force calculated data
  w5 = u16[] []  # Error String Number
  w6 = string[] []  # Error String Array
  w15 = TRUE  # Pass?
  w17 = sgl[] []  # Vent Force Raw Data
  n1 = Unbundle By Name("input cluster") -> ("Motion Status.Analog Data"=w1:sgl[][], "Store Data.Error Table"=w13:string[][], "Sequence State.Step Data String"=w14:string, "D in map.Abort Test"=w4:T20, "PLC Comms.PLC boolean read Tags"=w12:T25, "PLC Comms.PLC bool write Tags"=w11:T28, "Station Index"=w10:i32)  [unwired: 1 out]
  n2 = Unflatten From String(type=T1 {"Overall Min"=0.0, "Overall Max"=0.0, "Truncation Start"=0.0, "Truncation End"=0.0} ("Sun Shade Close Force"), binary string=w14) -> (value=w7:T1)  [unwired: 3 in, 2 out]
  "Sun Shade Close Force" <- w7
  n3 = Bundle("Error String Array"=w6, "Error String Number"=w5, "Vent Force Raw Data"=w17, "Sun Shade Close Force"=w7, "Pass?"=w15, "Error Table"=w13, "Vent Force calculated data"=w3, "Station Index"=w10, "PLC boolean read Tags"=w12, "PLC bool write Tags"=w11, "Abort Test"=w4, "Vent Force Data and Limits"=w2, "Analog Data"=w1) -> (w16:T46)  [unwired: 1 in]
  n4 = while {
    shift-right: [w19] -> _
    shift-left: string[] ["Init"] ("event queue out") -> [w24]
    shift-right: [w26] -> _
    shift-left: w16 -> [w27]
    tunnel: "input cluster" -> [w20]
    stop <- w22 continue-if-true
    n5 = call "EOL next state.vi"("Main State Cluster"=w20, "event queue in"=w24) -> ("Condition (Exit:F)"=w22:bool, "next event"=w21:string, "event queue out"=w23:string[])  [unwired: 5 in, 2 out]
    "State" <- w21
    n6 = Wait (ms)(milliseconds to wait=u32 5) -> ()  [unwired: 1 out]
    n7 = case shown="\"Get Force Data\"" w21 {
      selector: w21 -> [w29 _ _ _ _ _]
      tunnel: w23 -> [w33 _ w40 w59 w67 w75]
      tunnel: w27 -> [w28 w34 w44 w58 w69 w74]
      tunnel: [w28 w34 w43 w57 w68 w74] -> w26
      tunnel: [w33 string[] ["Get Force Data", "Calculate Force Data", "Check Force Data Limits", "Exit"] ("event queue out") w40 w59 w67 w75] -> w19
      frame "Error", Default {
        n8 = Concatenate Strings("Vent Anti-Pinch Test  Entered Error State - The Intended state was - " ("string"), w29) -> (w31:string)
        n9 = One Button Dialog(message=w31, button name ("OK")="OK") -> ()  [unwired: 1 out]
      }
      frame "Init" {
      }
      frame "Calculate Force Data" {
        n10 = Unbundle By Name(w44) -> ("Vent Force Raw Data"=w45:sgl[], "Sun Shade Close Force.Truncation Start"=w42:dbl, "Sun Shade Close Force.Truncation End"=w41:dbl)
        n11 = Multiply(x=w45, y="scaling factor") -> (x*y=w38:dbl[])
        n12 = Absolute Value(x=w38) -> (abs(x)=w37:dbl[])
        n13 = disable-structure shown="Enabled" {
          disable-tunnel: w42 -> [w51 _]
          disable-tunnel: w41 -> [w50 _]
          disable-tunnel: w37 -> [w47 w53]
          disable-tunnel: [w46 w52] -> w36
          frame Disabled {
            n14 = To Long Integer(number=w51) -> (32bit integer=w49:i32)
            n15 = To Long Integer(number=w50) -> (32bit integer=w48:i32)
            n16 = call "EOL Calculate Vent AP data.vi"("Truncation End"=w48, "Truncation Start"=w49, "Array Data"=w47) -> ("Vent Force calculated value"=w46:dbl)  [unwired: 8 in]
          }
          frame Enabled {
            n17 = Array Max & Min(array=w53) -> (max value=w52:dbl)  [unwired: 3 out]
          }
        }
        n18 = Bundle By Name(cluster=w44, "Vent Force Raw Data"=w37, "Vent Force calculated data"=w36) -> (w43:T46)
      }
      frame "Get Force Data" {
        n19 = Unbundle By Name(w58) -> ("Analog Data"=w54:sgl[][])
        n20 = Index Array(array=w54, index (col)=EOL_Analog_Input_Control."SW PS  Volage" ("Analog Control")) -> (element=w56:sgl[])  [unwired: 1 in]
        n21 = Bundle By Name(cluster=w58, "Vent Force Raw Data"=w56) -> (w57:T46)
      }
      frame "Check Force Data Limits" {
        n22 = Unbundle By Name(w69) -> ("Vent Force calculated data"=w66:dbl, "Sun Shade Close Force"=w62:T1, "Error Table"=w65:string[][], "Pass?"=w61:bool)
        n23 = call "EOL Check AP Vent Limits.vi"("Pass? In"=w61, "Error Table"=w65, "Sun Shade Close Force"=w62, "Vent Force Calculated Data"=w66) -> ("Error Table 2"=w63:string[][], "Vent Force Data and Limits"=w60:dbl[], "Pass?"=w64:bool)  [unwired: 5 in]
        n24 = Bundle By Name(cluster=w69, "Pass?"=w64, "Vent Force Data and Limits"=w60, "Error Table"=w63) -> (w68:T46)
      }
      frame "Exit" {
        n25 = Unbundle By Name(w74) -> ("Pass?"=→"Pass? Out":bool, "Error Table"=→"Error Table Out":string[][], "Vent Force Data and Limits"=→"Vent Force Data and Limits":dbl[], "Vent Force Raw Data"=→"Vent Force Raw Data":sgl[])
      }
    }
  }
